vi "Go.vi"(6 "assembly type":string, 8 "First?":bool, 9 "Timing Data":T1(array[cluster]), 10 "Control In":T2={"I-O.lvclass"=refnum, "Gantry"=refnum, "Dispenser"="COM1"}, 11 "Sensor Dispense in":refnum<class "Sensor Dispense.lvclass">) -> (2 "Control Out":T2={"I-O.lvclass"=refnum, "Gantry"=refnum, "Dispenser"="COM1"}, 3 "Sensor Dispense out":refnum<class "Sensor Dispense.lvclass">)   [LabVIEW 2021, in "Sensor Dispense.lvclass"]
uses:
  Sensor Dispense.lvclass
  C:/Users/HEP/Documents/GitHub/Gantry/UCSB-Gantry-HEP-main/Classes/Routine/Dispense/Dispense.lvclass
  Classes/Controller/Controllers.ctl
  Classes/Controller/I-O/I-O.lvclass
  C:/Program Files (x86)/Aerotech/A3200/LabVIEW/2010/Bin/Aerotech.A3200.dll
  Program Files (x86)/Aerotech/A3200/LabVIEW/2010/Bin/Aerotech.A3200.dll
  Sensor Dispense.lvclass/Sensor Dispense.ctl
  Classes/Controller/Motion/Motion.lvclass
  Classes/Controller/Dispenser/Dispenser.lvclass
  Classes/Controller/Motion/A3200/A3200.lvclass
  Classes/Controller/Controller.lvclass
panel:
  out "error out":errorcluster
  in  "error in (no error)":errorcluster
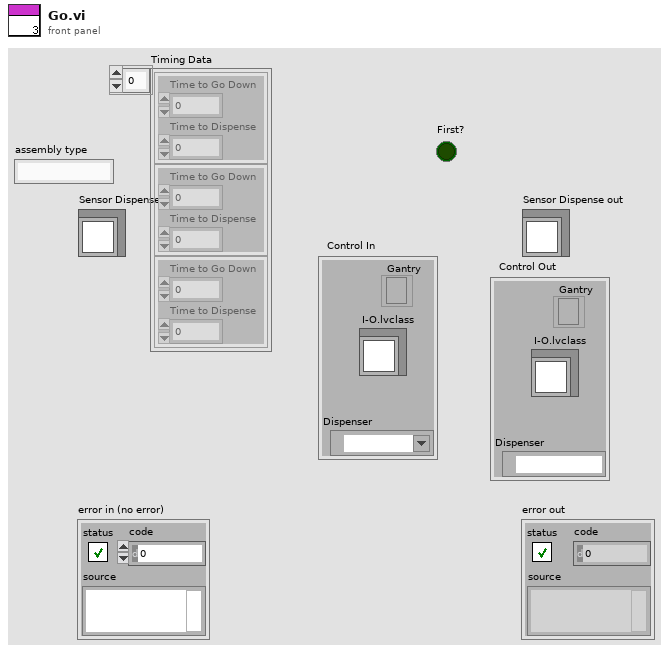
[diagram p1: front panel]
types:
  T1 = cluster{"Time to Go Down":i32, "Time to Dispense":i32}[]
  T2 = typedef "Controller.lvclass/Controllers.ctl" = cluster{"I-O.lvclass":refnum<class "I-O.lvclass">, "Gantry":refnum<k24>, "Dispenser":refnum<visa-resource-name>}
  T3 = cluster{"Endpoints":dbl[][], "Center":dbl[], "CW/CCW":dbl, "Dispense Type":enum16{"N-gon", "Square", "Arc", "Dot", "Line", "Circle"}}[]
  T4 = cluster{"Endpoints":dbl[][], "Center":dbl[], "CW/CCW":dbl, "Dispense Type":enum16{"N-gon", "Square", "Arc", "Dot", "Line", "Circle"}}
  T5 = enum16{"N-gon", "Square", "Arc", "Dot", "Line", "Circle"}
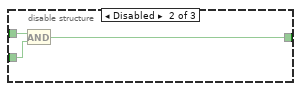
[diagram p3: hidden frame]
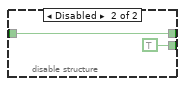
[diagram p4: hidden frame]
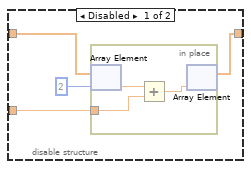
[diagram p6: hidden frame]
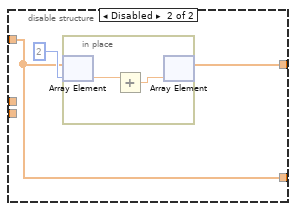
[diagram p7: hidden frame]
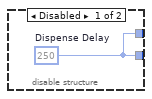
[diagram p9: hidden frame]
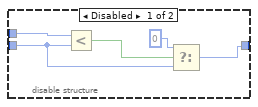
[diagram p10: hidden frame]
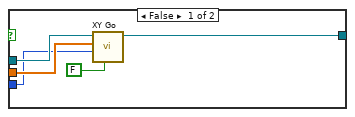
[diagram p11: hidden frame]
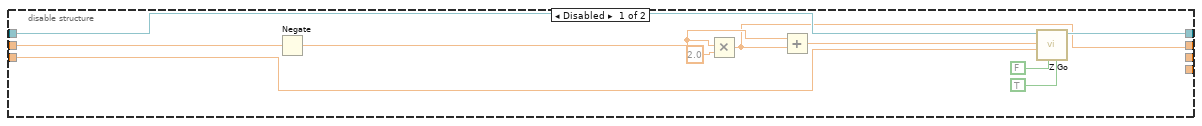
[diagram p12: hidden frame]
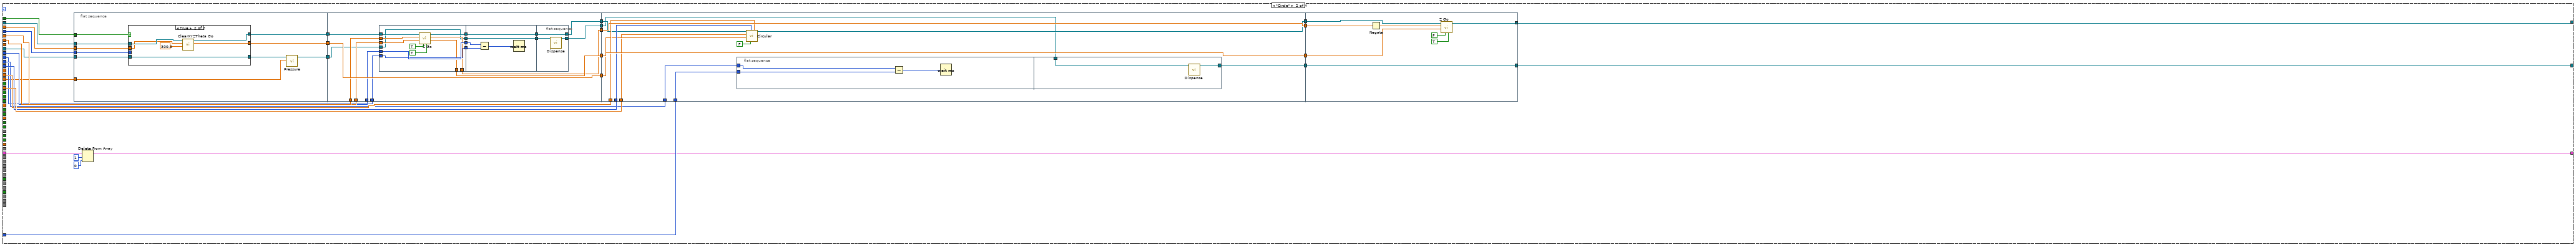
[diagram p14: hidden frame]
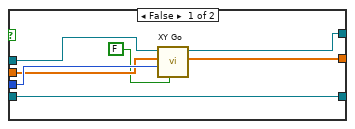
[diagram p15: hidden frame]
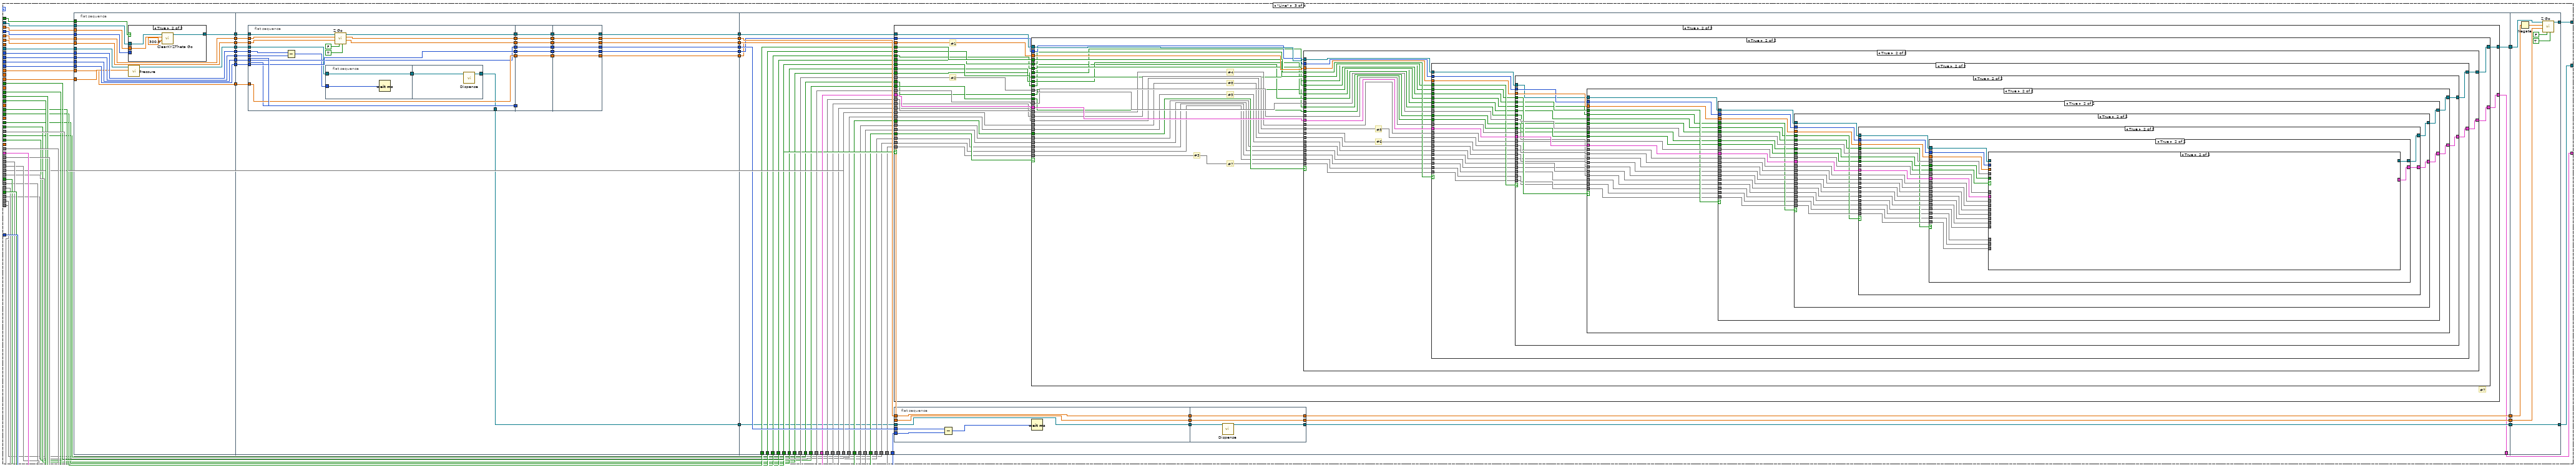
[diagram p16: hidden frame]
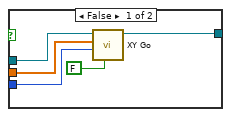
[diagram p17: hidden frame]
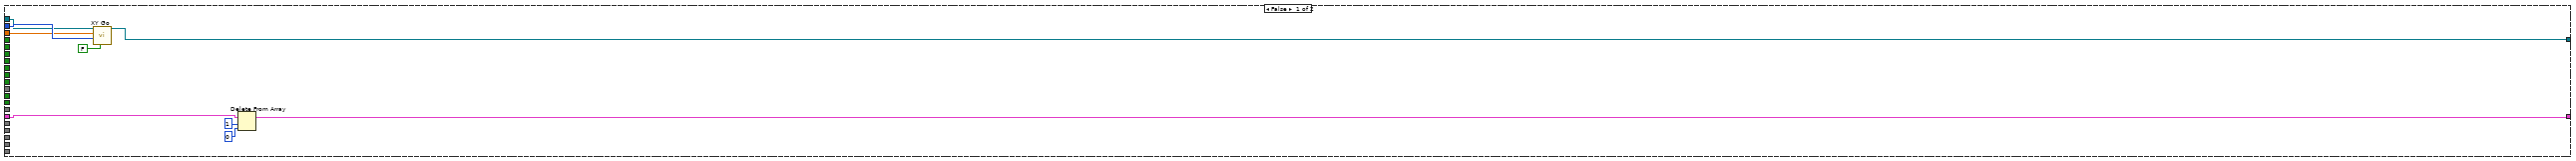
[diagram p18: hidden frame]
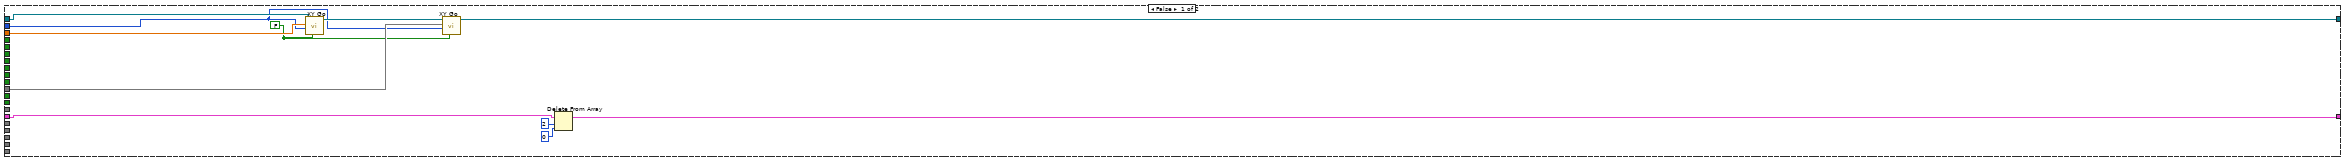
[diagram p19: hidden frame]
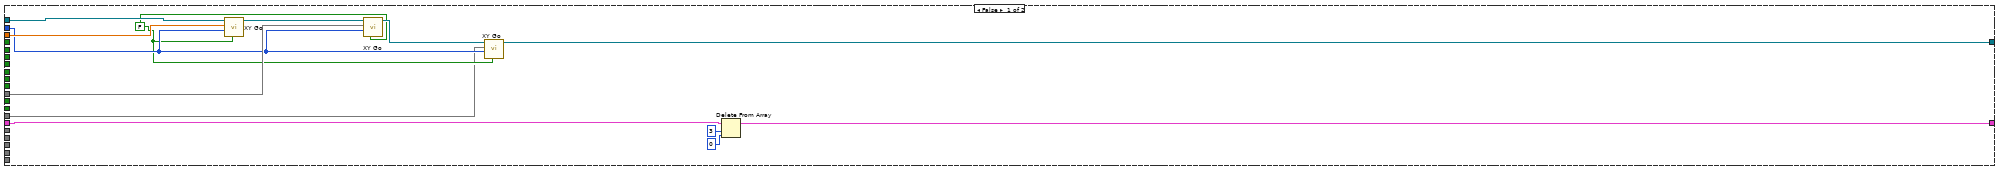
[diagram p20: hidden frame]
diagram:
  n1 = case shown="No Error" "error in (no error)" {
    selector: "error in (no error)" -> [w9 w1467]
    tunnel: "Sensor Dispense in" -> [w14 w1466]
    tunnel: [w13 w1466] -> w6
    tunnel: "Control In" -> [w12 w1465]
    tunnel: [w11 w1465] -> w4
    tunnel: [w10 w1467] -> w3
    tunnel: "First?" -> [w8 _]
    frame No Error {
      n2 = in-place {
        in-place-border: w14 -> [w27]
        in-place-border: [w26] -> w13
        in-place-border: w9 -> [w20]
        in-place-border: [w19] -> w10
        in-place-border: w8 -> [w15]
        n3 = in-place-cluster #1(w12) -> ("Gantry"=w28:refnum<k24>, "Dispenser"=w23:refnum<visa-resource-name>)
        n4 = Unbundle By Name(w27) -> ("Dispense Steps"=w24:T3, "Glue Speed"=w18:i32, "Move Speed"=w29:i32, "Line Pressure"=w16:dbl, "Dot Pressure"=w17:dbl)
        n5 = while {
          tunnel: w29 -> [w180]
          shift-right: [w174] -> w25
          shift-left: w28 -> [w43]
          tunnel: w18 -> [w179]
          shift-right: [w167] -> w26
          shift-left: w27 -> [w177]
          shift-right: [w169] -> w21
          shift-left: w23 -> [w172]
          tunnel: "Timing Data" -> [w171] mode=indexing
          shift-right: [w42] -> w19
          shift-left: w20 -> [w41]
          tunnel: w17 -> [w165]
          tunnel: w16 -> [w164]
          shift-right: [w128] -> _
          shift-left: w24 -> [w80]
          tunnel: w15 -> [w30]
          i -> [w176]
          stop <- w130 stop-if-true
          # "740 is good"
          # "compares 3 and 4"
          # "compares 2 and 3"
          # "Compares 1 and 2"
          # "#2"
          # "#3"
          # "#4"
          # "#3"
          # "1/11/23 - Originally 750"
          n6 = call "get Estop status.vi"("error in (no error)"=w41, "controller in"=w43) -> ("error out"=w42:errorcluster, "Estop?"=w40:bool, "controller out"=w36:refnum<k24>)  [unwired: 7 in]
          n7 = Equal To 0?(x=w176) -> (x = 0?=w31:bool)
          n8 = disable-structure shown="Enabled" {
            disable-tunnel: [w182 w185 w190] -> w32
            disable-tunnel: w31 -> [w182 w184 w191]
            disable-tunnel: w30 -> [w181 w183 w186]
            frame Disabled {
            }
            frame Disabled {
              n9 = And(x=w184, y=w183) -> (x .and. y?=w185:bool)
            }
            frame Enabled {
              n10 = disable-structure shown="Enabled" {
                disable-tunnel: [w194 TRUE ("protomodule? (T)")] -> w188
                disable-tunnel: [TRUE ("element") w195] -> w187
                disable-tunnel: w186 -> [_ w195]
                frame Enabled {
                  n11 = call "protomodule or module.vi"("assembly type"="assembly type") -> ("protomodule? (T)"=w194:bool)  [unwired: 10 in]
                }
                frame Disabled {
                }
              }
              n12 = Build Array(w191, w187, w188) -> (w189:bool[])
              n13 = And Array Elements(Boolean array=w189) -> (logical AND=w190:bool)
            }
          }
          n14 = Stop(stop? (T)=w40) -> ()
          n15 = Index Array(array=w80, index=6) -> (element=w123:T4)
          n16 = Index Array(array=w80, index=7) -> (element=w121:T4)
          n17 = Unbundle By Name(w123) -> ("Endpoints"=w122:dbl[][])  [unwired: 1 out]
          n18 = Unbundle By Name(w121) -> ("Endpoints"=w120:dbl[][])  [unwired: 1 out]
          n19 = Index Array(array=w122) -> (element #1=w105:dbl[], element #2=w46:dbl[])  [unwired: 4 in]
          n20 = Index Array(array=w120) -> (element #1=w99:dbl[], element #2=w78:dbl[])  [unwired: 4 in]
          n21 = Equal?(x=w46, y=w99) -> (x = y?=w100:bool[])
          n22 = Index Array(array=w80) -> (element=w160:T4)  [unwired: 1 in]
          n23 = Index Array(array=w100) -> (element #1=w98:bool, element #2=w97:bool)  [unwired: 2 in]
          n24 = And(x=w98, y=w97) -> (x .and. y?=w96:bool)
          n25 = Unbundle By Name(w160) -> ("Endpoints"=w151:dbl[][], "Center"=w173:dbl[], "Dispense Type"=w175:T5, "CW/CCW"=w178:dbl)
          n26 = property on="Property Node" class="Sensor Dispense.lvclass"(reference=w177) -> (reference out=w167:refnum<class "Sensor Dispense.lvclass">, "Z height"=w37:dbl, "Z speed"=w168:dbl, "Tip Height"=w34:dbl)  [unwired: 1 in, 1 out]
          n27 = Index Array(array=w151) -> (element #2=w150:dbl[])  [unwired: 4 in, 1 out]
          n28 = Index Array(array=w151) -> (element #1=w38:dbl[], element #2=w39:dbl[])  [unwired: 4 in]
          n29 = disable-structure shown="Enabled" {
            disable-tunnel: w36 -> [w203 w243]
            disable-tunnel: w38 -> [w197 w242]
            disable-tunnel: [w202 w243] -> w35
            disable-tunnel: w37 -> [w198 _]
            disable-tunnel: w32 -> [w201 _]
            disable-tunnel: w34 -> [w200 _]
            disable-tunnel: [w199 w242] -> w33
            frame Enabled {
              n30 = case shown="True" w201 {
                tunnel: w203 -> [w205 w214]
                tunnel: [w205 w209] -> w202
                tunnel: w200 -> [_ w206]
                tunnel: [w204 w210] -> w199
                tunnel: w198 -> [_ w208]
                tunnel: w197 -> [w204 w207]
                frame False {
                }
                frame True {
                  n31 = disable-structure shown="Enabled" {
                    disable-tunnel: [w220 w234] -> w213
                    disable-tunnel: [w219 w235] -> w210
                    disable-tunnel: w208 -> [w218 _]
                    disable-tunnel: w207 -> [w216 w235]
                    disable-tunnel: w206 -> [w215 _]
                    frame Enabled {
                      n32 = disable-structure shown="Enabled" {
                        disable-tunnel: [w224 w228] -> w219
                        disable-tunnel: w216 -> [w222 w228]
                        disable-tunnel: w215 -> [w221 _]
                        frame Disabled {
                          n33 = in-place {
                            in-place-border: w221 -> [w226]
                            n34 = in-place-array #2(w222, 2) -> (w227:dbl)
                            n35 = Add(x=w227, y=w226) -> (x+y=w225:dbl)
                            n36 = in-place-array #2(w225) -> (w224:dbl[])  [unwired: 1 out]
                          }
                        }
                        frame Enabled {
                        }
                      }
                      n37 = in-place {
                        in-place-border: w218 -> [w232]
                        in-place-border: w215 -> [w230]
                        n38 = in-place-array #3(w216, 2) -> (w233:dbl)
                        n39 = Negate(x=w230) -> (-x=w229:dbl)
                        n40 = Compound Arithmetic op=ADD(w233, w232, w229) -> (w231:dbl)
                        n41 = in-place-array #3(w231) -> (w220:dbl[])  [unwired: 1 out]
                      }
                    }
                    frame Disabled {
                      n42 = in-place {
                        n43 = in-place-array #4(w235, 2) -> (w238:dbl)
                        n44 = Add(x=w238) -> (x+y=w237:dbl)  [unwired: 1 in]
                        n45 = in-place-array #4(w237) -> (w234:dbl[])  [unwired: 1 out]
                      }
                    }
                  }
                  n46 = call "ClearXYZTheta Go.vi"("Speed"=300.0, "XYZTheta In"=w213, "Gantry In"=w214) -> ("error out"=w212:errorcluster, "Gantry Out"=w209:refnum<k24>)  [unwired: 6 in, 1 out]
                  n47 = while {
                    shift-right: [w239] -> _
                    shift-left: w212 -> [w240]
                    stop <- w241 stop-if-true
                    n48 = call "Prompt User for Input"("error in (no error)"=w240) -> ("Tip on component?"=w241:bool, "error out"=w239:errorcluster)  [unwired: 16 in, 1 out]
                  }
                }
              }
            }
            frame Disabled {
            }
          }
          n49 = Unbundle By Name(w171) -> ("Time to Go Down"=w170:i32, "Time to Dispense"=w162:i32)
          n50 = disable-structure shown="Enabled" {
            disable-tunnel: [w244 w248] -> w166
            disable-tunnel: [w244 w246] -> w163
            disable-tunnel: w162 -> [_ w247]
            frame Disabled {
              w244 = 250  # Dispense Delay
            }
            frame Enabled {
              w245 = 450  # End Dispense Delay
              w248 = 740  # Start Dispense Delay
              # "For arcs it is set to 250"
              # "525 - 1/23/2023"
              # "Originally 0"
              n51 = disable-structure shown="Enabled" {
                disable-tunnel: w247 -> [w253 _]
                disable-tunnel: [w250 w254] -> w246
                disable-tunnel: w245 -> [w249 w254]
                frame Disabled {
                  n52 = Less?(x=w253, y=w249) -> (x < y?=w252:bool)
                  n53 = Select(t=0, s=w252, f=w249) -> (s? t:f=w250:i32)
                }
                frame Enabled {
                }
              }
            }
          }
          n54 = Index Array(array=w80, index=2) -> (element=w157:T4)
          n55 = Index Array(array=w80, index=1) -> (element=w159:T4)
          n56 = Unbundle By Name(w157) -> ("Endpoints"=w154:dbl[][], "Center"=w135:dbl[])
          n57 = Unbundle By Name(w159) -> ("Endpoints"=w158:dbl[][], "Center"=w136:dbl[])
          n58 = Index Array(array=w80, index=3) -> (element=w156:T4)
          n59 = Unbundle By Name(w156) -> ("Endpoints"=w155:dbl[][], "Center"=w134:dbl[])
          n60 = Index Array(array=w154) -> (element #1=w148:dbl[], element #2=w44:dbl[])  [unwired: 4 in]
          n61 = Index Array(array=w158) -> (element #1=w149:dbl[], element #2=w137:dbl[])  [unwired: 4 in]
          n62 = Equal?(x=w150, y=w149) -> (x = y?=w146:bool[])
          n63 = Equal?(x=w137, y=w148) -> (x = y?=w143:bool[])
          n64 = Index Array(array=w155) -> (element #1=w147:dbl[], element #2=w45:dbl[])  [unwired: 4 in]
          n65 = Index Array(array=w80, index=10) -> (element=w89:T4)
          n66 = Index Array(array=w80, index=11) -> (element=w86:T4)
          n67 = Index Array(array=w80, index=12) -> (element=w83:T4)
          n68 = Equal?(x=w44, y=w147) -> (x = y?=w142:bool[])
          n69 = Index Array(array=w146) -> (element #1=w145:bool, element #2=w144:bool)  [unwired: 2 in]
          n70 = Index Array(array=w143) -> (element #1=w141:bool, element #2=w140:bool)  [unwired: 2 in]
          n71 = Index Array(array=w80, index=8) -> (element=w95:T4)
          n72 = Index Array(array=w80, index=9) -> (element=w92:T4)
          n73 = Index Array(array=w80, index=5) -> (element=w125:T4)
          n74 = Index Array(array=w80, index=4) -> (element=w127:T4)
          n75 = Unbundle By Name(w89) -> ("Endpoints"=w88:dbl[][])  [unwired: 1 out]
          n76 = Unbundle By Name(w86) -> ("Endpoints"=w85:dbl[][])  [unwired: 1 out]
          n77 = Unbundle By Name(w83) -> ("Endpoints"=w82:dbl[][])  [unwired: 1 out]
          n78 = Unbundle By Name(w95) -> ("Endpoints"=w94:dbl[][])  [unwired: 1 out]
          n79 = Unbundle By Name(w92) -> ("Endpoints"=w91:dbl[][])  [unwired: 1 out]
          n80 = Unbundle By Name(w125) -> ("Endpoints"=w124:dbl[][])  [unwired: 1 out]
          n81 = Unbundle By Name(w127) -> ("Endpoints"=w126:dbl[][])  [unwired: 1 out]
          n82 = And(x=w145, y=w144) -> (x .and. y?=w133:bool)
          n83 = Index Array(array=w142) -> (element #1=w139:bool, element #2=w138:bool)  [unwired: 2 in]
          n84 = And(x=w141, y=w140) -> (x .and. y?=w132:bool)
          n85 = And(x=w139, y=w138) -> (x .and. y?=w131:bool)
          n86 = Index Array(array=w88) -> (element #1=w67:dbl[], element #2=w61:dbl[])  [unwired: 4 in]
          n87 = Index Array(array=w85) -> (element #1=w60:dbl[], element #2=w55:dbl[])  [unwired: 4 in]
          n88 = Index Array(array=w82) -> (element #1=w54:dbl[], element #2=w49:dbl[])  [unwired: 4 in]
          n89 = Index Array(array=w94) -> (element #1=w79:dbl[], element #2=w72:dbl[])  [unwired: 4 in]
          n90 = Index Array(array=w91) -> (element #1=w73:dbl[], element #2=w66:dbl[])  [unwired: 4 in]
          n91 = Index Array(array=w124) -> (element #1=w110:dbl[], element #2=w48:dbl[])  [unwired: 4 in]
          n92 = Index Array(array=w126) -> (element #1=w115:dbl[], element #2=w47:dbl[])  [unwired: 4 in]
          n93 = Equal?(x=w61, y=w60) -> (x = y?=w59:bool[])
          n94 = Equal?(x=w48, y=w105) -> (x = y?=w104:bool[])
          n95 = Equal?(x=w55, y=w54) -> (x = y?=w53:bool[])
          n96 = Equal?(x=w66, y=w67) -> (x = y?=w65:bool[])
          n97 = Equal?(x=w72, y=w73) -> (x = y?=w71:bool[])
          n98 = Equal?(x=w47, y=w110) -> (x = y?=w109:bool[])
          n99 = Equal?(x=w78, y=w79) -> (x = y?=w77:bool[])
          n100 = Equal?(x=w45, y=w115) -> (x = y?=w114:bool[])
          n101 = Index Array(array=w59) -> (element #1=w58:bool, element #2=w57:bool)  [unwired: 2 in]
          n102 = Index Array(array=w104) -> (element #1=w103:bool, element #2=w102:bool)  [unwired: 2 in]
          n103 = Index Array(array=w53) -> (element #1=w52:bool, element #2=w51:bool)  [unwired: 2 in]
          n104 = Index Array(array=w65) -> (element #1=w64:bool, element #2=w63:bool)  [unwired: 2 in]
          n105 = Index Array(array=w71) -> (element #1=w70:bool, element #2=w69:bool)  [unwired: 2 in]
          n106 = Index Array(array=w109) -> (element #1=w108:bool, element #2=w107:bool)  [unwired: 2 in]
          n107 = Index Array(array=w77) -> (element #1=w76:bool, element #2=w75:bool)  [unwired: 2 in]
          n108 = Index Array(array=w114) -> (element #1=w113:bool, element #2=w112:bool)  [unwired: 2 in]
          n109 = And(x=w58, y=w57) -> (x .and. y?=w56:bool)
          n110 = And(x=w103, y=w102) -> (x .and. y?=w101:bool)
          n111 = And(x=w52, y=w51) -> (x .and. y?=w50:bool)
          n112 = And(x=w64, y=w63) -> (x .and. y?=w62:bool)
          n113 = And(x=w70, y=w69) -> (x .and. y?=w68:bool)
          n114 = And(x=w108, y=w107) -> (x .and. y?=w106:bool)
          n115 = And(x=w76, y=w75) -> (x .and. y?=w74:bool)
          n116 = And(x=w113, y=w112) -> (x .and. y?=w111:bool)
          n117 = case shown="\"Dot\", Default" w175 {
            tunnel: w173 -> [_ w408 _ w1258]
            tunnel: w35 -> [w284 w409 w501 w1264]
            tunnel: w180 -> [w269 w402 w559 w1263]
            tunnel: [w283 w412 w557 w1254] -> w174
            tunnel: w179 -> [_ w407 w551 w1257]
            tunnel: w178 -> [_ w406 _ w1256]
            tunnel: w168 -> [w277 w404 w548 w1259]
            tunnel: w37 -> [w278 w405 w549 w1260]
            tunnel: w31 -> [w285 w403 w498 w1265]
            tunnel: w172 -> [w276 w388 w554 w1250]
            tunnel: w170 -> [w274 w393 w552 w1262]
            tunnel: w162 -> [w279 w394 w550 w1255]
            tunnel: w166 -> [w280 w392 w553 w1261]
            tunnel: [w282 w389 w555 w1253] -> w169
            tunnel: w165 -> [w268 _ _ _]
            tunnel: w164 -> [_ w386 w531 w1249]
            tunnel: w163 -> [_ w385 w530 w1248]
            tunnel: w137 -> [_ _ w527 w1247]
            tunnel: w136 -> [_ _ _ w1246]
            tunnel: w135 -> [_ _ _ w1245]
            tunnel: w134 -> [_ _ _ w1244]
            tunnel: w45 -> [_ _ w522 w1243]
            tunnel: w133 -> [_ _ w525 w1242]
            tunnel: w132 -> [_ _ w524 w1241]
            tunnel: w131 -> [_ _ w523 w1240]
            tunnel: w80 -> [w260 w384 w528 w1239]
            tunnel: [w257 w381 w529 w1238] -> w128
            tunnel: w44 -> [_ _ w526 w1237]
            tunnel: w111 -> [_ _ w521 _]
            tunnel: w47 -> [_ _ w520 _]
            tunnel: w106 -> [_ _ w519 _]
            tunnel: w48 -> [_ _ w518 _]
            tunnel: w101 -> [_ _ w517 _]
            tunnel: w96 -> [_ _ w516 _]
            tunnel: w46 -> [_ _ w515 _]
            tunnel: w78 -> [_ _ w514 _]
            tunnel: w74 -> [_ _ w513 _]
            tunnel: w72 -> [_ _ w512 _]
            tunnel: w68 -> [_ _ w511 _]
            tunnel: w66 -> [_ _ w510 _]
            tunnel: w62 -> [_ _ w509 _]
            tunnel: w61 -> [_ _ w508 _]
            tunnel: w56 -> [_ _ w507 _]
            tunnel: w55 -> [_ _ w506 _]
            tunnel: w50 -> [_ _ w505 _]
            tunnel: w49 -> [_ _ w504 _]
            tunnel: w33 -> [w255 w380 w500 w1236]
            tunnel: w39 -> [_ _ w499 w1235]
            frame "Dot", Default {
              n118 = flat-sequence {
                tunnel: w285 -> [w286]
                tunnel: w284 -> [w297]
                tunnel: w255 -> [w296]
                tunnel: [w295] -> w281
                tunnel: w280 -> [w292]
                tunnel: w279 -> [_]
                tunnel: w278 -> [w294]
                tunnel: w277 -> [w291]
                tunnel: w276 -> [w289]
                tunnel: [w294] -> w275
                tunnel: w274 -> [w293]
                tunnel: [w293] -> w273
                tunnel: [w292] -> w272
                tunnel: [w288] -> w271
                tunnel: [w291] -> w270
                tunnel: w269 -> [w290]
                tunnel: w268 -> [w287]
                tunnel: [w324] -> w265
                tunnel: w281 -> [w323]
                tunnel: [w320] -> w264
                tunnel: w275 -> [w319]
                tunnel: w273 -> [w318]
                tunnel: w272 -> [w317]
                tunnel: w271 -> [w316]
                tunnel: w270 -> [w313]
                tunnel: [w311] -> w263
                tunnel: [w310] -> w262
                tunnel: w265 -> [w352]
                tunnel: w264 -> [w351]
                tunnel: w263 -> [w350]
                tunnel: w262 -> [w349]
                tunnel: [w353] -> w267
                tunnel: [w352] -> w266
                tunnel: [w347] -> w261
                tunnel: [w348] -> w256
                tunnel: [w367] -> w282
                tunnel: [w370] -> w283
                tunnel: w267 -> [w371]
                tunnel: w266 -> [w367]
                tunnel: w261 -> [w369]
                tunnel: w256 -> [w368]
                frame #0 {
                  n119 = case shown="True" w286 {
                    tunnel: w297 -> [w302 w306]
                    tunnel: [w301 w305] -> w295
                    tunnel: w296 -> [w300 w304]
                    tunnel: w290 -> [w299 _]
                    frame False {
                      n120 = call "XY Go.vi"("return immediately"=FALSE, "Speed"=w299, "XY In"=w300, "Gantry In"=w302) -> ("Gantry Out"=w301:refnum<k24>)  [unwired: 5 in, 2 out]
                    }
                    frame True {
                      n121 = call "ClearXYZTheta Go.vi"("Speed"=300.0, "XYZTheta In"=w304, "Gantry In"=w306) -> ("Gantry Out"=w305:refnum<k24>)  [unwired: 6 in, 2 out]
                    }
                  }
                  n122 = call "Pressure.vi"("Pressure"=w287, "VISA resource name"=w289) -> ("VISA resource name out"=w288:refnum<visa-resource-name>)  [unwired: 8 in, 1 out]
                }
                frame #1 {
                  n123 = flat-sequence {
                    tunnel: w323 -> [w333]
                    tunnel: [w332] -> w321
                    tunnel: w319 -> [w326]
                    tunnel: w316 -> [w330]
                    tunnel: [w330] -> w315
                    tunnel: w313 -> [w329]
                    tunnel: [w328] -> w308
                    tunnel: [w325] -> w307
                    tunnel: [w340] -> w322
                    tunnel: w321 -> [w340]
                    tunnel: w318 -> [w339]
                    tunnel: w317 -> [w335]
                    tunnel: w315 -> [w338]
                    tunnel: [w338] -> w314
                    tunnel: [w337] -> w312
                    tunnel: [w336] -> w309
                    tunnel: w308 -> [w336]
                    tunnel: w307 -> [w337]
                    tunnel: [w346] -> w324
                    tunnel: w322 -> [w345]
                    tunnel: [w345] -> w320
                    tunnel: w314 -> [w344]
                    tunnel: w312 -> [w342]
                    tunnel: [w342] -> w311
                    tunnel: [w341] -> w310
                    tunnel: w309 -> [w341]
                    frame #0 {
                      n124 = call "Z Go.vi"("Increment"=TRUE, "Return Immediately"=TRUE, "Speed In"=w329, "Position In"=w326, "Gantry In"=w333) -> ("Speed Out"=w328:dbl, "Position Out"=w325:dbl, "Gantry Out"=w332:refnum<k24>)  [unwired: 3 in, 1 out]
                    }
                    frame #1 {
                      n125 = Subtract(x=w339, y=w335) -> (x-y=w334:i32)
                      n126 = Wait (ms)(milliseconds to wait=w334) -> ()  [unwired: 1 out]
                    }
                    frame #2 {
                      n127 = call "Dispense.vi"("Dispenser In"=w344) -> ("Dispenser Out"=w343:refnum<visa-resource-name>)  [unwired: 9 in, 1 out]
                      n128 = call "Dispense.vi"("Dispenser In"=w343) -> ("Dispenser Out"=w346:refnum<visa-resource-name>)  [unwired: 9 in, 1 out]
                    }
                  }
                }
                frame #2 {
                  n129 = disable-structure shown="Enabled" {
                    disable-tunnel: [w363 w366] -> w353
                    disable-tunnel: w351 -> [w362 w366]
                    disable-tunnel: w350 -> [w361 w364]
                    disable-tunnel: w349 -> [w358 w365]
                    disable-tunnel: [w354 _] -> _
                    disable-tunnel: [_ w365] -> w348
                    disable-tunnel: [_ w364] -> w347
                    frame Disabled {
                      n130 = Negate(x=w361) -> (-x=w356:dbl)
                      n131 = Multiply(x=w356, y=2.0) -> (x*y=w354:dbl)
                      n132 = Add(x=w356, y=w354) -> (x+y=w357:dbl)
                      n133 = call "Z Go.vi"("Increment"=TRUE, "Return Immediately"=FALSE, "Speed In"=w358, "Position In"=w357, "Gantry In"=w362) -> ("Gantry Out"=w363:refnum<k24>)  [unwired: 3 in, 3 out]
                    }
                    frame Enabled {
                    }
                  }
                }
                frame #3 {
                  n134 = disable-structure shown="Enabled" {
                    disable-tunnel: w371 -> [w378 w379]
                    disable-tunnel: [w377 w379] -> w370
                    disable-tunnel: w369 -> [w372 _]
                    disable-tunnel: w368 -> [w373 _]
                    frame Enabled {
                      n135 = Negate(x=w372) -> (-x=w376:dbl)
                      n136 = call "Z Go.vi"("Increment"=TRUE, "Return Immediately"=FALSE, "Speed In"=w373, "Position In"=w376, "Gantry In"=w378) -> ("Gantry Out"=w377:refnum<k24>)  [unwired: 3 in, 3 out]
                    }
                    frame Disabled {
                    }
                  }
                }
              }
              n137 = Delete From Array(array=w260, length=1, index=0) -> (array with subset deleted=w257:T3)  [unwired: 1 out]
            }
            frame "Circle" {
              n138 = flat-sequence {
                tunnel: [w421] -> w411
                tunnel: w409 -> [w422]
                tunnel: w403 -> [w413]
                tunnel: w402 -> [w420]
                tunnel: [w419] -> w400
                tunnel: w380 -> [w418]
                tunnel: w388 -> [w417]
                tunnel: [w415] -> w387
                tunnel: w386 -> [w414]
                tunnel: w405 -> [w445]
                tunnel: w404 -> [w446]
                tunnel: [w452] -> w401
                tunnel: [w443] -> w399
                tunnel: [w444] -> w398
                tunnel: w400 -> [w452]
                tunnel: w411 -> [w442]
                tunnel: [w451] -> w395
                tunnel: w393 -> [w450]
                tunnel: w392 -> [w449]
                tunnel: [w439] -> w391
                tunnel: w387 -> [w438]
                tunnel: [w474] -> w410
                tunnel: [w484] -> w397
                tunnel: [w483] -> w396
                tunnel: w394 -> [w482]
                tunnel: w395 -> [w472]
                tunnel: w401 -> [w477]
                tunnel: w399 -> [w484]
                tunnel: w398 -> [w483]
                tunnel: w406 -> [w480]
                tunnel: w407 -> [w478]
                tunnel: w408 -> [w476]
                tunnel: w391 -> [w475]
                tunnel: [w481] -> w390
                tunnel: w385 -> [w473]
                tunnel: [w495] -> w412
                tunnel: w410 -> [w496]
                tunnel: w397 -> [w497]
                tunnel: w396 -> [w494]
                tunnel: w390 -> [w493]
                tunnel: [w493] -> w389
                frame #0 {
                  n139 = case shown="True" w413 {
                    tunnel: w422 -> [w429 w435]
                    tunnel: [w428 w434] -> w421
                    tunnel: w420 -> [w427 _]
                    tunnel: [w426 w432] -> w419
                    tunnel: w418 -> [w425 w433]
                    tunnel: w417 -> [w424 w431]
                    tunnel: [w424 w431] -> w416
                    frame False {
                      n140 = call "XY Go.vi"("return immediately"=FALSE, "Speed"=w427, "XY In"=w425, "Gantry In"=w429) -> ("XY Out"=w426:dbl[], "Gantry Out"=w428:refnum<k24>)  [unwired: 5 in, 1 out]
                    }
                    frame True {
                      n141 = call "ClearXYZTheta Go.vi"("Speed"=300.0, "XYZTheta In"=w433, "Gantry In"=w435) -> ("XYZTheta Out"=w432:dbl[], "Gantry Out"=w434:refnum<k24>)  [unwired: 6 in, 1 out]
                    }
                  }
                  n142 = call "Pressure.vi"("Pressure"=w414, "VISA resource name"=w416) -> ("VISA resource name out"=w415:refnum<visa-resource-name>)  [unwired: 8 in, 1 out]
                }
                frame #1 {
                  n143 = flat-sequence {
                    tunnel: w449 -> [w462]
                    tunnel: w450 -> [w463]
                    tunnel: [w463] -> w448
                    tunnel: [w462] -> w447
                    tunnel: w446 -> [w461]
                    tunnel: w445 -> [w460]
                    tunnel: [w459] -> w444
                    tunnel: [w458] -> w443
                    tunnel: w442 -> [w457]
                    tunnel: [w456] -> w441
                    tunnel: w438 -> [w454]
                    tunnel: [w454] -> w437
                    tunnel: w448 -> [w468]
                    tunnel: w447 -> [w467]
                    tunnel: w441 -> [w466]
                    tunnel: [w466] -> w440
                    tunnel: w437 -> [w465]
                    tunnel: [w465] -> w436
                    tunnel: [w471] -> w451
                    tunnel: w440 -> [w470]
                    tunnel: [w470] -> w439
                    tunnel: w436 -> [w469]
                    frame #0 {
                      n144 = call "Z Go.vi"("Increment"=TRUE, "Return Immediately"=TRUE ("return immediately"), "Speed In"=w461, "Position In"=w460, "Gantry In"=w457) -> ("Speed Out"=w459:dbl, "Position Out"=w458:dbl, "Gantry Out"=w456:refnum<k24>)  [unwired: 3 in, 1 out]
                    }
                    frame #1 {
                      n145 = Subtract(x=w468, y=w467) -> (x-y=w464:i32)
                      n146 = Wait (ms)(milliseconds to wait=w464) -> ()  [unwired: 1 out]
                    }
                    frame #2 {
                      n147 = call "Dispense.vi"("Dispenser In"=w469) -> ("Dispenser Out"=w471:refnum<visa-resource-name>)  [unwired: 9 in, 1 out]
                    }
                  }
                }
                frame #2 {
                  n148 = flat-sequence {
                    tunnel: w482 -> [w487]
                    tunnel: w473 -> [w485]
                    tunnel: [w489] -> w481
                    tunnel: w472 -> [w488]
                    frame #0 {
                      n149 = Subtract(x=w487, y=w485) -> (x-y=w486:i32)
                      n150 = Wait (ms)(milliseconds to wait=w486) -> ()  [unwired: 1 out]
                    }
                    frame #1 {
                      n151 = call "Dispense.vi"("Dispenser In"=w488) -> ("Dispenser Out"=w489:refnum<visa-resource-name>)  [unwired: 9 in, 1 out]
                    }
                  }
                  n152 = call "Circular.vi"("Direction"=w480, "return immediately"=FALSE, "Speed"=w478, "XY End"=w477, "XY Center"=w476, "Gantry In"=w475) -> ("Gantry Out"=w474:refnum<k24>)  [unwired: 4 in, 1 out]
                }
                frame #3 {
                  n153 = Negate(x=w497) -> (-x=w492:dbl)
                  n154 = call "Z Go.vi"("Increment"=TRUE, "Return Immediately"=FALSE, "Speed In"=w494, "Position In"=w492, "Gantry In"=w496) -> ("Gantry Out"=w495:refnum<k24>)  [unwired: 3 in, 3 out]
                }
              }
              n155 = Delete From Array(array=w384, length=1, index=0) -> (array with subset deleted=w381:T3)  [unwired: 1 out]
            }
            frame "Line" {
              n156 = flat-sequence {
                tunnel: w501 -> [w574]
                tunnel: w559 -> [w573]
                tunnel: [w572] -> w558
                tunnel: w554 -> [w565]
                tunnel: w553 -> [w568]
                tunnel: w552 -> [w569]
                tunnel: w551 -> [w567]
                tunnel: w550 -> [w566]
                tunnel: w549 -> [w571]
                tunnel: w548 -> [w570]
                tunnel: [w571] -> w547
                tunnel: [w570] -> w546
                tunnel: [w569] -> w544
                tunnel: [w568] -> w543
                tunnel: [w564] -> w542
                tunnel: [w561] -> w540
                tunnel: [w567] -> w538
                tunnel: [w566] -> w536
                tunnel: w531 -> [w563]
                tunnel: w500 -> [w562]
                tunnel: w499 -> [w561]
                tunnel: w498 -> [w560]
                tunnel: w558 -> [w607]
                tunnel: w547 -> [w606]
                tunnel: w546 -> [w605]
                tunnel: [w602] -> w545
                tunnel: w544 -> [w599]
                tunnel: w543 -> [w600]
                tunnel: w542 -> [w601]
                tunnel: [w613] -> w541
                tunnel: w540 -> [w612]
                tunnel: [w611] -> w539
                tunnel: w538 -> [w610]
                tunnel: [w608] -> w537
                tunnel: w536 -> [w609]
                tunnel: [w604] -> w533
                tunnel: [w603] -> w503
                tunnel: [w584] -> w502
                tunnel: [w687] -> w556
                tunnel: w545 -> [w676]
                tunnel: w541 -> [w677]
                tunnel: w539 -> [w678]
                tunnel: w537 -> [w685]
                tunnel: [w675] -> w535
                tunnel: [w684] -> w534
                tunnel: w533 -> [w682]
                tunnel: [w681] -> w532
                tunnel: w530 -> [w674]
                tunnel: [w673] -> w529
                tunnel: w528 -> [w672]
                tunnel: w527 -> [w671]
                tunnel: w526 -> [w670]
                tunnel: w525 -> [w669]
                tunnel: w524 -> [w668]
                tunnel: w523 -> [w667]
                tunnel: w522 -> [w666]
                tunnel: w521 -> [w665]
                tunnel: w520 -> [w664]
                tunnel: w519 -> [w663]
                tunnel: w518 -> [w662]
                tunnel: w517 -> [w661]
                tunnel: w516 -> [w660]
                tunnel: w515 -> [w659]
                tunnel: w514 -> [w658]
                tunnel: w513 -> [w657]
                tunnel: w512 -> [w656]
                tunnel: w511 -> [w655]
                tunnel: w510 -> [w654]
                tunnel: w509 -> [w653]
                tunnel: w508 -> [w652]
                tunnel: w507 -> [w651]
                tunnel: w506 -> [w650]
                tunnel: w505 -> [w649]
                tunnel: w504 -> [w648]
                tunnel: w503 -> [w679]
                tunnel: w502 -> [w647]
                tunnel: [w1234] -> w557
                tunnel: w556 -> [w1233]
                tunnel: [w1233] -> w555
                tunnel: w535 -> [w1232]
                tunnel: w534 -> [w1231]
                tunnel: w532 -> [w1229]
                frame #0 {
                  n157 = case shown="True" w560 {
                    tunnel: w574 -> [w579 w583]
                    tunnel: w573 -> [w578 _]
                    tunnel: [w577 w582] -> w572
                    tunnel: w562 -> [w576 w581]
                    frame False {
                      n158 = call "XY Go.vi"("return immediately"=FALSE, "Speed"=w578, "XY In"=w576, "Gantry In"=w579) -> ("Gantry Out"=w577:refnum<k24>)  [unwired: 5 in, 2 out]
                    }
                    frame True {
                      n159 = call "ClearXYZTheta Go.vi"("Speed"=300.0, "XYZTheta In"=w581, "Gantry In"=w583) -> ("Gantry Out"=w582:refnum<k24>)  [unwired: 6 in, 2 out]
                    }
                  }
                  n160 = call "Pressure.vi"("Pressure"=w563, "VISA resource name"=w565) -> ("VISA resource name out"=w564:refnum<visa-resource-name>)  [unwired: 8 in, 1 out]
                }
                frame #1 {
                  n161 = flat-sequence {
                    tunnel: w599 -> [w622]
                    tunnel: w600 -> [w614]
                    tunnel: w612 -> [w621]
                    tunnel: w610 -> [w620]
                    tunnel: w609 -> [w619]
                    tunnel: w607 -> [w630]
                    tunnel: w606 -> [w629]
                    tunnel: w605 -> [w628]
                    tunnel: w601 -> [w616]
                    tunnel: [w622] -> w598
                    tunnel: [w614] -> w597
                    tunnel: [w621] -> w596
                    tunnel: [w620] -> w595
                    tunnel: [w619] -> w594
                    tunnel: [w625] -> w593
                    tunnel: [w624] -> w592
                    tunnel: [w623] -> w591
                    tunnel: [w617] -> w584
                    tunnel: w598 -> [_]
                    tunnel: w597 -> [_]
                    tunnel: w596 -> [w640]
                    tunnel: w595 -> [w639]
                    tunnel: w594 -> [w638]
                    tunnel: w593 -> [w637]
                    tunnel: w592 -> [w636]
                    tunnel: w591 -> [w635]
                    tunnel: [w640] -> w590
                    tunnel: [w639] -> w589
                    tunnel: [w638] -> w588
                    tunnel: [w637] -> w587
                    tunnel: [w636] -> w586
                    tunnel: [w635] -> w585
                    tunnel: [w646] -> w613
                    tunnel: [w645] -> w611
                    tunnel: [w644] -> w608
                    tunnel: [w643] -> w604
                    tunnel: [w642] -> w603
                    tunnel: [w641] -> w602
                    tunnel: w590 -> [w646]
                    tunnel: w589 -> [w645]
                    tunnel: w588 -> [w644]
                    tunnel: w587 -> [w643]
                    tunnel: w586 -> [w642]
                    tunnel: w585 -> [w641]
                    frame #0 {
                      n162 = Subtract(x=w622, y=w614) -> (x-y=w618:i32)
                      n163 = flat-sequence {
                        tunnel: w618 -> [w632]
                        tunnel: w616 -> [w631]
                        tunnel: [w631] -> w615
                        tunnel: [w634] -> w617
                        tunnel: w615 -> [w633]
                        frame #0 {
                          n164 = Wait (ms)(milliseconds to wait=w632) -> ()  [unwired: 1 out]
                        }
                        frame #1 {
                          n165 = call "Dispense.vi"("Dispenser In"=w633) -> ("Dispenser Out"=w634:refnum<visa-resource-name>)  [unwired: 9 in, 1 out]
                        }
                      }
                      n166 = call "Z Go.vi"("Increment"=TRUE ("Return Immediately"), "Return Immediately"=FALSE ("Increment"), "Speed In"=w628, "Position In"=w629, "Gantry In"=w630) -> ("Speed Out"=w624:dbl, "Position Out"=w625:dbl, "Gantry Out"=w623:refnum<k24>)  [unwired: 3 in, 1 out]
                    }
                    frame #1 {
                    }
                    frame #2 {
                    }
                  }
                }
                frame #2 {
                  n167 = case shown="True" w669 {
                    tunnel: w678 -> [w696 w721]
                    tunnel: w677 -> [w695 w724]
                    tunnel: w676 -> [w694 w723]
                    tunnel: [w693 w720] -> w675
                    tunnel: [w690 w719] -> w673
                    tunnel: w672 -> [w691 w725]
                    tunnel: w671 -> [_ w722]
                    tunnel: w670 -> [_ w718]
                    tunnel: w668 -> [_ w717]
                    tunnel: w667 -> [_ w716]
                    tunnel: w666 -> [_ w715]
                    tunnel: w665 -> [_ w714]
                    tunnel: w664 -> [_ w713]
                    tunnel: w663 -> [_ w712]
                    tunnel: w662 -> [_ w711]
                    tunnel: w661 -> [_ w710]
                    tunnel: w660 -> [_ w709]
                    tunnel: w659 -> [_ w708]
                    tunnel: w658 -> [_ w707]
                    tunnel: w657 -> [_ w706]
                    tunnel: w656 -> [_ w705]
                    tunnel: w655 -> [_ w704]
                    tunnel: w654 -> [_ w703]
                    tunnel: w653 -> [_ w702]
                    tunnel: w652 -> [_ w701]
                    tunnel: w651 -> [_ w700]
                    tunnel: w650 -> [_ w699]
                    tunnel: w649 -> [_ w698]
                    tunnel: w648 -> [_ w697]
                    frame False {
                      n168 = call "XY Go.vi"("return immediately"=FALSE, "Speed"=w696, "XY In"=w695, "Gantry In"=w694) -> ("Gantry Out"=w693:refnum<k24>)  [unwired: 5 in, 2 out]
                      n169 = Delete From Array(array=w691, length=1, index=0) -> (array with subset deleted=w690:T3)  [unwired: 1 out]
                    }
                    frame True {
                      # "#7"
                      # "#2"
                      # "#1"
                      n170 = case shown="True" w717 {
                        tunnel: w725 -> [w736 w764]
                        tunnel: w724 -> [w733 w762]
                        tunnel: w723 -> [w732 w760]
                        tunnel: w722 -> [w730 w761]
                        tunnel: w721 -> [w729 w758]
                        tunnel: [w728 w759] -> w720
                        tunnel: [w727 w763] -> w719
                        tunnel: w718 -> [_ w757]
                        tunnel: w716 -> [_ w756]
                        tunnel: w715 -> [_ w755]
                        tunnel: w714 -> [_ w754]
                        tunnel: w713 -> [_ w753]
                        tunnel: w712 -> [_ w752]
                        tunnel: w711 -> [_ w751]
                        tunnel: w710 -> [_ w750]
                        tunnel: w709 -> [_ w749]
                        tunnel: w708 -> [_ w748]
                        tunnel: w707 -> [_ w747]
                        tunnel: w706 -> [_ w746]
                        tunnel: w705 -> [_ w745]
                        tunnel: w704 -> [_ w744]
                        tunnel: w703 -> [_ w743]
                        tunnel: w702 -> [_ w742]
                        tunnel: w701 -> [_ w741]
                        tunnel: w700 -> [_ w740]
                        tunnel: w699 -> [_ w739]
                        tunnel: w698 -> [_ w738]
                        tunnel: w697 -> [_ w737]
                        frame False {
                          w726 = FALSE ("return immediately")
                          n171 = call "XY Go.vi"("return immediately"=w726, "Speed"=w729, "XY In"=w733, "Gantry In"=w732) -> ("Gantry Out"=w731:refnum<k24>)  [unwired: 5 in, 2 out]
                          n172 = call "XY Go.vi"("return immediately"=w726, "Speed"=w729, "XY In"=w730, "Gantry In"=w731) -> ("Gantry Out"=w728:refnum<k24>)  [unwired: 5 in, 2 out]
                          n173 = Delete From Array(array=w736, length=2, index=0) -> (array with subset deleted=w727:T3)  [unwired: 1 out]
                        }
                        frame True {
                          # "#9"
                          # "#8"
                          # "#3"
                          # "#4"
                          # "#7"
                          n174 = case shown="True" w756 {
                            tunnel: w764 -> [w777 w798]
                            tunnel: [w774 w797] -> w763
                            tunnel: w762 -> [w773 w804]
                            tunnel: w761 -> [w772 w803]
                            tunnel: w760 -> [w771 w800]
                            tunnel: [w768 w799] -> w759
                            tunnel: w758 -> [w767 w801]
                            tunnel: w757 -> [w765 w802]
                            tunnel: w755 -> [_ w796]
                            tunnel: w754 -> [_ w795]
                            tunnel: w753 -> [_ w794]
                            tunnel: w752 -> [_ w793]
                            tunnel: w751 -> [_ w792]
                            tunnel: w750 -> [_ w791]
                            tunnel: w749 -> [_ w790]
                            tunnel: w748 -> [_ w789]
                            tunnel: w747 -> [_ w788]
                            tunnel: w746 -> [_ w787]
                            tunnel: w745 -> [_ w786]
                            tunnel: w744 -> [_ w785]
                            tunnel: w743 -> [_ w784]
                            tunnel: w742 -> [_ w783]
                            tunnel: w741 -> [_ w782]
                            tunnel: w740 -> [_ w781]
                            tunnel: w739 -> [_ w780]
                            tunnel: w738 -> [_ w779]
                            tunnel: w737 -> [_ w778]
                            frame False {
                              w766 = FALSE ("return immediately")
                              n175 = call "XY Go.vi"("return immediately"=w766, "Speed"=w767, "XY In"=w773, "Gantry In"=w771) -> ("Gantry Out"=w770:refnum<k24>)  [unwired: 5 in, 2 out]
                              n176 = call "XY Go.vi"("return immediately"=w766, "Speed"=w767, "XY In"=w772, "Gantry In"=w770) -> ("Gantry Out"=w769:refnum<k24>)  [unwired: 5 in, 2 out]
                              n177 = call "XY Go.vi"("return immediately"=w766, "Speed"=w767, "XY In"=w765, "Gantry In"=w769) -> ("Gantry Out"=w768:refnum<k24>)  [unwired: 5 in, 2 out]
                              n178 = Delete From Array(array=w777, length=3, index=0) -> (array with subset deleted=w774:T3)  [unwired: 1 out]
                            }
                            frame True {
                              # "#5"
                              # "#6"
                              n179 = case shown="True" w795 {
                                tunnel: w804 -> [w818 w842]
                                tunnel: w803 -> [w817 w841]
                                tunnel: w802 -> [w816 w840]
                                tunnel: w801 -> [w815 w838]
                                tunnel: w800 -> [w814 w837]
                                tunnel: [w810 w836] -> w799
                                tunnel: w798 -> [w807 w844]
                                tunnel: [w806 w843] -> w797
                                tunnel: w796 -> [w805 w839]
                                tunnel: w794 -> [_ w835]
                                tunnel: w793 -> [_ w834]
                                tunnel: w792 -> [_ w819]
                                tunnel: w791 -> [_ w833]
                                tunnel: w790 -> [_ w832]
                                tunnel: w789 -> [_ w831]
                                tunnel: w788 -> [_ w830]
                                tunnel: w787 -> [_ w829]
                                tunnel: w786 -> [_ w828]
                                tunnel: w785 -> [_ w827]
                                tunnel: w784 -> [_ w826]
                                tunnel: w783 -> [_ w825]
                                tunnel: w782 -> [_ w824]
                                tunnel: w781 -> [_ w823]
                                tunnel: w780 -> [_ w822]
                                tunnel: w779 -> [_ w821]
                                tunnel: w778 -> [_ w820]
                                frame False {
                                n180 = call "XY Go.vi"("Speed"=w815, "XY In"=w818, "Gantry In"=w814) -> ("Gantry Out"=w813:refnum<k24>)  [unwired: 6 in, 2 out]
                                n181 = call "XY Go.vi"("Speed"=w815, "XY In"=w817, "Gantry In"=w813) -> ("Gantry Out"=w812:refnum<k24>)  [unwired: 6 in, 2 out]
                                n182 = call "XY Go.vi"("Speed"=w815, "XY In"=w816, "Gantry In"=w812) -> ("Gantry Out"=w811:refnum<k24>)  [unwired: 6 in, 2 out]
                                n183 = call "XY Go.vi"("Speed"=w815, "XY In"=w805, "Gantry In"=w811) -> ("Gantry Out"=w810:refnum<k24>)  [unwired: 6 in, 2 out]
                                n184 = Delete From Array(array=w807, length=4, index=0) -> (array with subset deleted=w806:T3)  [unwired: 1 out]
                                }
                                frame True {
                                n185 = case shown="True" w834 {
                                tunnel: w844 -> [w860 w885]
                                tunnel: [w859 w884] -> w843
                                tunnel: w842 -> [w856 w883]
                                tunnel: w841 -> [w855 w882]
                                tunnel: w840 -> [w854 w880]
                                tunnel: w839 -> [w853 w879]
                                tunnel: w838 -> [w852 w878]
                                tunnel: w837 -> [w851 w877]
                                tunnel: [w846 w876] -> w836
                                tunnel: w835 -> [w845 w881]
                                tunnel: w819 -> [_ w875]
                                tunnel: w833 -> [_ w874]
                                tunnel: w832 -> [_ w873]
                                tunnel: w831 -> [_ w872]
                                tunnel: w830 -> [_ w871]
                                tunnel: w829 -> [_ w870]
                                tunnel: w828 -> [_ w869]
                                tunnel: w827 -> [_ w868]
                                tunnel: w826 -> [_ w867]
                                tunnel: w825 -> [_ w866]
                                tunnel: w824 -> [_ w865]
                                tunnel: w823 -> [_ w864]
                                tunnel: w822 -> [_ w863]
                                tunnel: w821 -> [_ w862]
                                tunnel: w820 -> [_ w861]
                                frame False {
                                n186 = call "XY Go.vi"("Speed"=w852, "XY In"=w856, "Gantry In"=w851) -> ("Gantry Out"=w850:refnum<k24>)  [unwired: 6 in, 2 out]
                                n187 = call "XY Go.vi"("Speed"=w852, "XY In"=w855, "Gantry In"=w850) -> ("Gantry Out"=w849:refnum<k24>)  [unwired: 6 in, 2 out]
                                n188 = call "XY Go.vi"("Speed"=w852, "XY In"=w854, "Gantry In"=w849) -> ("Gantry Out"=w848:refnum<k24>)  [unwired: 6 in, 2 out]
                                n189 = call "XY Go.vi"("Speed"=w852, "XY In"=w853, "Gantry In"=w848) -> ("Gantry Out"=w847:refnum<k24>)  [unwired: 6 in, 2 out]
                                n190 = call "XY Go.vi"("Speed"=w852, "XY In"=w845, "Gantry In"=w847) -> ("Gantry Out"=w846:refnum<k24>)  [unwired: 6 in, 2 out]
                                n191 = Delete From Array(array=w860, length=5, index=0) -> (array with subset deleted=w859:T3)  [unwired: 1 out]
                                }
                                frame True {
                                n192 = case shown="True" w874 {
                                tunnel: w885 -> [w901 w927]
                                tunnel: [w900 w926] -> w884
                                tunnel: w883 -> [w899 w925]
                                tunnel: w882 -> [w898 w924]
                                tunnel: w881 -> [w888 w923]
                                tunnel: w880 -> [w886 w922]
                                tunnel: w879 -> [w887 w920]
                                tunnel: w878 -> [w897 w919]
                                tunnel: w877 -> [w896 w918]
                                tunnel: [w890 w917] -> w876
                                tunnel: w875 -> [w889 w921]
                                tunnel: w873 -> [_ w916]
                                tunnel: w872 -> [_ w915]
                                tunnel: w871 -> [_ w914]
                                tunnel: w870 -> [_ w913]
                                tunnel: w869 -> [_ w912]
                                tunnel: w868 -> [_ w911]
                                tunnel: w867 -> [_ w910]
                                tunnel: w866 -> [_ w909]
                                tunnel: w865 -> [_ w908]
                                tunnel: w864 -> [_ w907]
                                tunnel: w863 -> [_ w906]
                                tunnel: w862 -> [_ w905]
                                tunnel: w861 -> [_ w904]
                                frame False {
                                n193 = call "XY Go.vi"("Speed"=w897, "XY In"=w899, "Gantry In"=w896) -> ("Gantry Out"=w895:refnum<k24>)  [unwired: 6 in, 2 out]
                                n194 = call "XY Go.vi"("Speed"=w897, "XY In"=w898, "Gantry In"=w895) -> ("Gantry Out"=w894:refnum<k24>)  [unwired: 6 in, 2 out]
                                n195 = call "XY Go.vi"("Speed"=w897, "XY In"=w886, "Gantry In"=w894) -> ("Gantry Out"=w893:refnum<k24>)  [unwired: 6 in, 2 out]
                                n196 = call "XY Go.vi"("Speed"=w897, "XY In"=w887, "Gantry In"=w893) -> ("Gantry Out"=w892:refnum<k24>)  [unwired: 6 in, 2 out]
                                n197 = call "XY Go.vi"("Speed"=w897, "XY In"=w888, "Gantry In"=w892) -> ("Gantry Out"=w891:refnum<k24>)  [unwired: 6 in, 2 out]
                                n198 = call "XY Go.vi"("Speed"=w897, "XY In"=w889, "Gantry In"=w891) -> ("Gantry Out"=w890:refnum<k24>)  [unwired: 6 in, 2 out]
                                n199 = Delete From Array(array=w901, length=6, index=0) -> (array with subset deleted=w900:T3)  [unwired: 1 out]
                                }
                                frame True {
                                n200 = case shown="True" w916 {
                                tunnel: w927 -> [w945 w960]
                                tunnel: [w944 w959] -> w926
                                tunnel: w925 -> [w943 w970]
                                tunnel: w924 -> [w942 w969]
                                tunnel: w923 -> [w928 w968]
                                tunnel: w922 -> [w930 w967]
                                tunnel: w921 -> [w929 w966]
                                tunnel: w920 -> [w931 w965]
                                tunnel: w919 -> [w941 w963]
                                tunnel: w918 -> [w940 w962]
                                tunnel: [w933 w961] -> w917
                                tunnel: w915 -> [w932 w964]
                                tunnel: w914 -> [_ w958]
                                tunnel: w913 -> [_ w957]
                                tunnel: w912 -> [_ w956]
                                tunnel: w911 -> [_ w955]
                                tunnel: w910 -> [_ w954]
                                tunnel: w909 -> [_ w953]
                                tunnel: w908 -> [_ w952]
                                tunnel: w907 -> [_ w951]
                                tunnel: w906 -> [_ w950]
                                tunnel: w905 -> [_ w949]
                                tunnel: w904 -> [_ w948]
                                frame False {
                                n201 = call "XY Go.vi"("Speed"=w941, "XY In"=w943, "Gantry In"=w940) -> ("Gantry Out"=w939:refnum<k24>)  [unwired: 6 in, 2 out]
                                n202 = call "XY Go.vi"("Speed"=w941, "XY In"=w942, "Gantry In"=w939) -> ("Gantry Out"=w938:refnum<k24>)  [unwired: 6 in, 2 out]
                                n203 = call "XY Go.vi"("Speed"=w941, "XY In"=w930, "Gantry In"=w938) -> ("Gantry Out"=w937:refnum<k24>)  [unwired: 6 in, 2 out]
                                n204 = call "XY Go.vi"("Speed"=w941, "XY In"=w931, "Gantry In"=w937) -> ("Gantry Out"=w936:refnum<k24>)  [unwired: 6 in, 2 out]
                                n205 = call "XY Go.vi"("Speed"=w941, "XY In"=w928, "Gantry In"=w936) -> ("Gantry Out"=w935:refnum<k24>)  [unwired: 6 in, 2 out]
                                n206 = call "XY Go.vi"("Speed"=w941, "XY In"=w929, "Gantry In"=w935) -> ("Gantry Out"=w934:refnum<k24>)  [unwired: 6 in, 2 out]
                                n207 = call "XY Go.vi"("Speed"=w941, "XY In"=w932, "Gantry In"=w934) -> ("Gantry Out"=w933:refnum<k24>)  [unwired: 6 in, 2 out]
                                n208 = Delete From Array(array=w945, length=7, index=0) -> (array with subset deleted=w944:T3)  [unwired: 1 out]
                                }
                                frame True {
                                n209 = case shown="True" w957 {
                                tunnel: w970 -> [w992 w1012]
                                tunnel: w969 -> [w991 w1011]
                                tunnel: w968 -> [w972 w1010]
                                tunnel: w967 -> [w974 w1009]
                                tunnel: w966 -> [w971 w1008]
                                tunnel: w965 -> [w973 w1007]
                                tunnel: w964 -> [w990 w1006]
                                tunnel: w963 -> [w989 w1004]
                                tunnel: w962 -> [w988 w1003]
                                tunnel: [w980 w1002] -> w961
                                tunnel: w960 -> [w977 w1014]
                                tunnel: [w976 w1013] -> w959
                                tunnel: w958 -> [w975 w1005]
                                tunnel: w956 -> [_ w1001]
                                tunnel: w955 -> [_ w1000]
                                tunnel: w954 -> [_ w999]
                                tunnel: w953 -> [_ w998]
                                tunnel: w952 -> [_ w997]
                                tunnel: w951 -> [_ w996]
                                tunnel: w950 -> [_ w995]
                                tunnel: w949 -> [_ w994]
                                tunnel: w948 -> [_ w993]
                                frame False {
                                n210 = call "XY Go.vi"("Speed"=w989, "XY In"=w992, "Gantry In"=w988) -> ("Gantry Out"=w987:refnum<k24>)  [unwired: 6 in, 2 out]
                                n211 = call "XY Go.vi"("Speed"=w989, "XY In"=w991, "Gantry In"=w987) -> ("Gantry Out"=w986:refnum<k24>)  [unwired: 6 in, 2 out]
                                n212 = call "XY Go.vi"("Speed"=w989, "XY In"=w974, "Gantry In"=w986) -> ("Gantry Out"=w985:refnum<k24>)  [unwired: 6 in, 2 out]
                                n213 = call "XY Go.vi"("Speed"=w989, "XY In"=w973, "Gantry In"=w985) -> ("Gantry Out"=w984:refnum<k24>)  [unwired: 6 in, 2 out]
                                n214 = call "XY Go.vi"("Speed"=w989, "XY In"=w972, "Gantry In"=w984) -> ("Gantry Out"=w983:refnum<k24>)  [unwired: 6 in, 2 out]
                                n215 = call "XY Go.vi"("Speed"=w989, "XY In"=w971, "Gantry In"=w983) -> ("Gantry Out"=w982:refnum<k24>)  [unwired: 6 in, 2 out]
                                n216 = call "XY Go.vi"("Speed"=w989, "XY In"=w990, "Gantry In"=w982) -> ("Gantry Out"=w981:refnum<k24>)  [unwired: 6 in, 2 out]
                                n217 = call "XY Go.vi"("Speed"=w989, "XY In"=w975, "Gantry In"=w981) -> ("Gantry Out"=w980:refnum<k24>)  [unwired: 6 in, 2 out]
                                n218 = Delete From Array(array=w977, length=8, index=0) -> (array with subset deleted=w976:T3)  [unwired: 1 out]
                                }
                                frame True {
                                n219 = case shown="True" w1000 {
                                tunnel: w1014 -> [w1038 w1059]
                                tunnel: [w1037 w1058] -> w1013
                                tunnel: w1012 -> [w1034 w1057]
                                tunnel: w1011 -> [w1033 w1056]
                                tunnel: w1010 -> [w1018 w1055]
                                tunnel: w1009 -> [w1017 w1054]
                                tunnel: w1008 -> [w1016 w1053]
                                tunnel: w1007 -> [w1015 w1052]
                                tunnel: w1006 -> [w1032 w1051]
                                tunnel: w1005 -> [w1031 w1050]
                                tunnel: w1004 -> [w1030 w1048]
                                tunnel: w1003 -> [w1029 w1047]
                                tunnel: [w1020 w1046] -> w1002
                                tunnel: w1001 -> [w1019 w1049]
                                tunnel: w999 -> [_ w1045]
                                tunnel: w998 -> [_ w1044]
                                tunnel: w997 -> [_ w1043]
                                tunnel: w996 -> [_ w1042]
                                tunnel: w995 -> [_ w1041]
                                tunnel: w994 -> [_ w1040]
                                tunnel: w993 -> [_ w1039]
                                frame False {
                                n220 = call "XY Go.vi"("Speed"=w1030, "XY In"=w1034, "Gantry In"=w1029) -> ("Gantry Out"=w1028:refnum<k24>)  [unwired: 6 in, 2 out]
                                n221 = call "XY Go.vi"("Speed"=w1030, "XY In"=w1033, "Gantry In"=w1028) -> ("Gantry Out"=w1027:refnum<k24>)  [unwired: 6 in, 2 out]
                                n222 = call "XY Go.vi"("Speed"=w1030, "XY In"=w1017, "Gantry In"=w1027) -> ("Gantry Out"=w1026:refnum<k24>)  [unwired: 6 in, 2 out]
                                n223 = call "XY Go.vi"("Speed"=w1030, "XY In"=w1015, "Gantry In"=w1026) -> ("Gantry Out"=w1025:refnum<k24>)  [unwired: 6 in, 2 out]
                                n224 = call "XY Go.vi"("Speed"=w1030, "XY In"=w1018, "Gantry In"=w1025) -> ("Gantry Out"=w1024:refnum<k24>)  [unwired: 6 in, 2 out]
                                n225 = call "XY Go.vi"("Speed"=w1030, "XY In"=w1016, "Gantry In"=w1024) -> ("Gantry Out"=w1023:refnum<k24>)  [unwired: 6 in, 2 out]
                                n226 = call "XY Go.vi"("Speed"=w1030, "XY In"=w1032, "Gantry In"=w1023) -> ("Gantry Out"=w1022:refnum<k24>)  [unwired: 6 in, 2 out]
                                n227 = call "XY Go.vi"("Speed"=w1030, "XY In"=w1031, "Gantry In"=w1022) -> ("Gantry Out"=w1021:refnum<k24>)  [unwired: 6 in, 2 out]
                                n228 = call "XY Go.vi"("Speed"=w1030, "XY In"=w1019, "Gantry In"=w1021) -> ("Gantry Out"=w1020:refnum<k24>)  [unwired: 6 in, 2 out]
                                n229 = Delete From Array(array=w1038, length=9, index=0) -> (array with subset deleted=w1037:T3)  [unwired: 1 out]
                                }
                                frame True {
                                n230 = case shown="True" w1044 {
                                tunnel: w1059 -> [w1085 w1105]
                                tunnel: [w1082 w1104] -> w1058
                                tunnel: w1057 -> [w1081 w1101]
                                tunnel: w1056 -> [w1080 w1100]
                                tunnel: w1055 -> [w1063 w1099]
                                tunnel: w1054 -> [w1062 w1098]
                                tunnel: w1053 -> [w1061 w1097]
                                tunnel: w1052 -> [w1060 w1096]
                                tunnel: w1051 -> [w1079 w1095]
                                tunnel: w1050 -> [w1078 w1094]
                                tunnel: w1049 -> [w1077 w1093]
                                tunnel: w1048 -> [w1076 w1091]
                                tunnel: w1047 -> [w1075 w1103]
                                tunnel: [w1065 w1102] -> w1046
                                tunnel: w1045 -> [w1064 w1092]
                                tunnel: w1043 -> [_ w1090]
                                tunnel: w1042 -> [_ w1089]
                                tunnel: w1041 -> [_ w1088]
                                tunnel: w1040 -> [_ w1087]
                                tunnel: w1039 -> [_ w1086]
                                frame False {
                                n231 = call "XY Go.vi"("Speed"=w1076, "XY In"=w1081, "Gantry In"=w1075) -> ("Gantry Out"=w1074:refnum<k24>)  [unwired: 6 in, 2 out]
                                n232 = Delete From Array(array=w1085, length=10, index=0) -> (array with subset deleted=w1082:T3)  [unwired: 1 out]
                                n233 = call "XY Go.vi"("Speed"=w1076, "XY In"=w1080, "Gantry In"=w1074) -> ("Gantry Out"=w1073:refnum<k24>)  [unwired: 6 in, 2 out]
                                n234 = call "XY Go.vi"("Speed"=w1076, "XY In"=w1062, "Gantry In"=w1073) -> ("Gantry Out"=w1072:refnum<k24>)  [unwired: 6 in, 2 out]
                                n235 = call "XY Go.vi"("Speed"=w1076, "XY In"=w1060, "Gantry In"=w1072) -> ("Gantry Out"=w1071:refnum<k24>)  [unwired: 6 in, 2 out]
                                n236 = call "XY Go.vi"("Speed"=w1076, "XY In"=w1063, "Gantry In"=w1071) -> ("Gantry Out"=w1070:refnum<k24>)  [unwired: 6 in, 2 out]
                                n237 = call "XY Go.vi"("Speed"=w1076, "XY In"=w1061, "Gantry In"=w1070) -> ("Gantry Out"=w1069:refnum<k24>)  [unwired: 6 in, 2 out]
                                n238 = call "XY Go.vi"("Speed"=w1076, "XY In"=w1079, "Gantry In"=w1069) -> ("Gantry Out"=w1068:refnum<k24>)  [unwired: 6 in, 2 out]
                                n239 = call "XY Go.vi"("Speed"=w1076, "XY In"=w1078, "Gantry In"=w1068) -> ("Gantry Out"=w1067:refnum<k24>)  [unwired: 6 in, 2 out]
                                n240 = call "XY Go.vi"("Speed"=w1076, "XY In"=w1077, "Gantry In"=w1067) -> ("Gantry Out"=w1066:refnum<k24>)  [unwired: 6 in, 2 out]
                                n241 = call "XY Go.vi"("Speed"=w1076, "XY In"=w1064, "Gantry In"=w1066) -> ("Gantry Out"=w1065:refnum<k24>)  [unwired: 6 in, 2 out]
                                }
                                frame True {
                                n242 = case shown="True" w1089 {
                                tunnel: w1105 -> [w1133 w1152]
                                tunnel: [w1130 w1151] -> w1104
                                tunnel: w1103 -> [w1129 w1139]
                                tunnel: [w1118 w1138] -> w1102
                                tunnel: w1101 -> [w1117 w1150]
                                tunnel: w1100 -> [w1116 w1149]
                                tunnel: w1099 -> [w1110 w1148]
                                tunnel: w1098 -> [w1108 w1147]
                                tunnel: w1097 -> [w1109 w1146]
                                tunnel: w1096 -> [w1111 w1145]
                                tunnel: w1095 -> [w1115 w1144]
                                tunnel: w1094 -> [w1114 w1143]
                                tunnel: w1093 -> [w1106 w1142]
                                tunnel: w1092 -> [w1107 w1141]
                                tunnel: w1091 -> [w1113 w1134]
                                tunnel: w1090 -> [w1112 w1140]
                                tunnel: w1088 -> [_ w1137]
                                tunnel: w1087 -> [_ w1136]
                                tunnel: w1086 -> [_ w1135]
                                frame False {
                                n243 = call "XY Go.vi"("Speed"=w1113, "XY In"=w1117, "Gantry In"=w1129) -> ("Gantry Out"=w1128:refnum<k24>)  [unwired: 6 in, 2 out]
                                n244 = Delete From Array(array=w1133, length=11, index=0) -> (array with subset deleted=w1130:T3)  [unwired: 1 out]
                                n245 = call "XY Go.vi"("Speed"=w1113, "XY In"=w1116, "Gantry In"=w1128) -> ("Gantry Out"=w1127:refnum<k24>)  [unwired: 6 in, 2 out]
                                n246 = call "XY Go.vi"("Speed"=w1113, "XY In"=w1108, "Gantry In"=w1127) -> ("Gantry Out"=w1126:refnum<k24>)  [unwired: 6 in, 2 out]
                                n247 = call "XY Go.vi"("Speed"=w1113, "XY In"=w1111, "Gantry In"=w1126) -> ("Gantry Out"=w1125:refnum<k24>)  [unwired: 6 in, 2 out]
                                n248 = call "XY Go.vi"("Speed"=w1113, "XY In"=w1110, "Gantry In"=w1125) -> ("Gantry Out"=w1124:refnum<k24>)  [unwired: 6 in, 2 out]
                                n249 = call "XY Go.vi"("Speed"=w1113, "XY In"=w1109, "Gantry In"=w1124) -> ("Gantry Out"=w1123:refnum<k24>)  [unwired: 6 in, 2 out]
                                n250 = call "XY Go.vi"("Speed"=w1113, "XY In"=w1115, "Gantry In"=w1123) -> ("Gantry Out"=w1122:refnum<k24>)  [unwired: 6 in, 2 out]
                                n251 = call "XY Go.vi"("Speed"=w1113, "XY In"=w1114, "Gantry In"=w1122) -> ("Gantry Out"=w1121:refnum<k24>)  [unwired: 6 in, 2 out]
                                n252 = call "XY Go.vi"("Speed"=w1113, "XY In"=w1106, "Gantry In"=w1121) -> ("Gantry Out"=w1120:refnum<k24>)  [unwired: 6 in, 2 out]
                                n253 = call "XY Go.vi"("Speed"=w1113, "XY In"=w1107, "Gantry In"=w1120) -> ("Gantry Out"=w1119:refnum<k24>)  [unwired: 6 in, 2 out]
                                n254 = call "XY Go.vi"("Speed"=w1113, "XY In"=w1112, "Gantry In"=w1119) -> ("Gantry Out"=w1118:refnum<k24>)  [unwired: 6 in, 2 out]
                                }
                                frame True {
                                n255 = case shown="True" w1136 {
                                tunnel: w1152 -> [w1181 w1214]
                                tunnel: [w1180 w1213] -> w1151
                                tunnel: w1150 -> [w1179 w1212]
                                tunnel: w1149 -> [w1178 w1211]
                                tunnel: w1148 -> [w1155 w1186]
                                tunnel: w1147 -> [w1153 w1184]
                                tunnel: w1146 -> [w1154 w1187]
                                tunnel: w1145 -> [w1156 w1185]
                                tunnel: w1144 -> [w1177 w1210]
                                tunnel: w1143 -> [w1176 w1209]
                                tunnel: w1142 -> [w1175 w1208]
                                tunnel: w1141 -> [w1174 w1207]
                                tunnel: w1140 -> [w1173 w1206]
                                tunnel: w1139 -> [w1172 w1203]
                                tunnel: [w1160 w1190] -> w1138
                                tunnel: w1137 -> [w1159 w1205]
                                tunnel: w1135 -> [_ w1204]
                                tunnel: w1134 -> [w1157 w1189]
                                frame False {
                                w1158 = FALSE
                                n256 = Delete From Array(array=w1181, length=12, index=0) -> (array with subset deleted=w1180:T3)  [unwired: 1 out]
                                n257 = call "XY Go.vi"("return immediately"=w1158, "Speed"=w1157, "XY In"=w1179, "Gantry In"=w1172) -> ("Gantry Out"=w1171:refnum<k24>)  [unwired: 5 in, 2 out]
                                n258 = call "XY Go.vi"("return immediately"=w1158, "Speed"=w1157, "XY In"=w1178, "Gantry In"=w1171) -> ("Gantry Out"=w1170:refnum<k24>)  [unwired: 5 in, 2 out]
                                n259 = call "XY Go.vi"("return immediately"=w1158, "Speed"=w1157, "XY In"=w1153, "Gantry In"=w1170) -> ("Gantry Out"=w1169:refnum<k24>)  [unwired: 5 in, 2 out]
                                n260 = call "XY Go.vi"("return immediately"=w1158, "Speed"=w1157, "XY In"=w1156, "Gantry In"=w1169) -> ("Gantry Out"=w1168:refnum<k24>)  [unwired: 5 in, 2 out]
                                n261 = call "XY Go.vi"("return immediately"=w1158, "Speed"=w1157, "XY In"=w1155, "Gantry In"=w1168) -> ("Gantry Out"=w1167:refnum<k24>)  [unwired: 5 in, 2 out]
                                n262 = call "XY Go.vi"("return immediately"=w1158, "Speed"=w1157, "XY In"=w1154, "Gantry In"=w1167) -> ("Gantry Out"=w1166:refnum<k24>)  [unwired: 5 in, 2 out]
                                n263 = call "XY Go.vi"("return immediately"=w1158, "Speed"=w1157, "XY In"=w1177, "Gantry In"=w1166) -> ("Gantry Out"=w1165:refnum<k24>)  [unwired: 5 in, 2 out]
                                n264 = call "XY Go.vi"("return immediately"=w1158, "Speed"=w1157, "XY In"=w1176, "Gantry In"=w1165) -> ("Gantry Out"=w1164:refnum<k24>)  [unwired: 5 in, 2 out]
                                n265 = call "XY Go.vi"("return immediately"=w1158, "Speed"=w1157, "XY In"=w1175, "Gantry In"=w1164) -> ("Gantry Out"=w1163:refnum<k24>)  [unwired: 5 in, 2 out]
                                n266 = call "XY Go.vi"("return immediately"=w1158, "Speed"=w1157, "XY In"=w1174, "Gantry In"=w1163) -> ("Gantry Out"=w1162:refnum<k24>)  [unwired: 5 in, 2 out]
                                n267 = call "XY Go.vi"("return immediately"=w1158, "Speed"=w1157, "XY In"=w1173, "Gantry In"=w1162) -> ("Gantry Out"=w1161:refnum<k24>)  [unwired: 5 in, 2 out]
                                n268 = call "XY Go.vi"("return immediately"=w1158, "Speed"=w1157, "XY In"=w1159, "Gantry In"=w1161) -> ("Gantry Out"=w1160:refnum<k24>)  [unwired: 5 in, 2 out]
                                }
                                frame True {
                                w1188 = FALSE
                                n269 = Delete From Array(array=w1214, length=13, index=0) -> (array with subset deleted=w1213:T3)  [unwired: 1 out]
                                n270 = call "XY Go.vi"("return immediately"=w1188, "Speed"=w1189, "XY In"=w1212, "Gantry In"=w1203) -> ("Gantry Out"=w1202:refnum<k24>)  [unwired: 5 in, 2 out]
                                n271 = call "XY Go.vi"("return immediately"=w1188, "Speed"=w1189, "XY In"=w1211, "Gantry In"=w1202) -> ("Gantry Out"=w1201:refnum<k24>)  [unwired: 5 in, 2 out]
                                n272 = call "XY Go.vi"("return immediately"=w1188, "Speed"=w1189, "XY In"=w1184, "Gantry In"=w1201) -> ("Gantry Out"=w1200:refnum<k24>)  [unwired: 5 in, 2 out]
                                n273 = call "XY Go.vi"("return immediately"=w1188, "Speed"=w1189, "XY In"=w1185, "Gantry In"=w1200) -> ("Gantry Out"=w1199:refnum<k24>)  [unwired: 5 in, 2 out]
                                n274 = call "XY Go.vi"("return immediately"=w1188, "Speed"=w1189, "XY In"=w1186, "Gantry In"=w1199) -> ("Gantry Out"=w1198:refnum<k24>)  [unwired: 5 in, 2 out]
                                n275 = call "XY Go.vi"("return immediately"=w1188, "Speed"=w1189, "XY In"=w1187, "Gantry In"=w1198) -> ("Gantry Out"=w1197:refnum<k24>)  [unwired: 5 in, 2 out]
                                n276 = call "XY Go.vi"("return immediately"=w1188, "Speed"=w1189, "XY In"=w1210, "Gantry In"=w1197) -> ("Gantry Out"=w1196:refnum<k24>)  [unwired: 5 in, 2 out]
                                n277 = call "XY Go.vi"("return immediately"=w1188, "Speed"=w1189, "XY In"=w1209, "Gantry In"=w1196) -> ("Gantry Out"=w1195:refnum<k24>)  [unwired: 5 in, 2 out]
                                n278 = call "XY Go.vi"("return immediately"=w1188, "Speed"=w1189, "XY In"=w1208, "Gantry In"=w1195) -> ("Gantry Out"=w1194:refnum<k24>)  [unwired: 5 in, 2 out]
                                n279 = call "XY Go.vi"("return immediately"=w1188, "Speed"=w1189, "XY In"=w1207, "Gantry In"=w1194) -> ("Gantry Out"=w1193:refnum<k24>)  [unwired: 5 in, 2 out]
                                n280 = call "XY Go.vi"("return immediately"=w1188, "Speed"=w1189, "XY In"=w1206, "Gantry In"=w1193) -> ("Gantry Out"=w1192:refnum<k24>)  [unwired: 5 in, 2 out]
                                n281 = call "XY Go.vi"("return immediately"=w1188, "Speed"=w1189, "XY In"=w1205, "Gantry In"=w1192) -> ("Gantry Out"=w1191:refnum<k24>)  [unwired: 5 in, 2 out]
                                n282 = call "XY Go.vi"("return immediately"=w1188, "Speed"=w1189, "XY In"=w1204, "Gantry In"=w1191) -> ("Gantry Out"=w1190:refnum<k24>)  [unwired: 5 in, 2 out]
                                }
                                }
                                }
                                }
                                }
                                }
                                }
                                }
                                }
                                }
                                }
                                }
                                }
                                }
                                }
                                }
                                }
                              }
                            }
                          }
                        }
                      }
                    }
                  }
                  n283 = flat-sequence {
                    tunnel: [w1217] -> w686
                    tunnel: [w1221] -> w683
                    tunnel: [w1220] -> w680
                    tunnel: w685 -> [w1222]
                    tunnel: w682 -> [w1221]
                    tunnel: w679 -> [w1220]
                    tunnel: w674 -> [w1218]
                    tunnel: w647 -> [w1217]
                    tunnel: [w1226] -> w687
                    tunnel: w686 -> [w1225]
                    tunnel: [w1224] -> w684
                    tunnel: w683 -> [w1224]
                    tunnel: [w1223] -> w681
                    tunnel: w680 -> [w1223]
                    frame #0 {
                      n284 = Subtract(x=w1222, y=w1218) -> (x-y=w1219:i32)
                      n285 = Wait (ms)(milliseconds to wait=w1219) -> ()  [unwired: 1 out]
                    }
                    frame #1 {
                      n286 = call "Dispense.vi"("Dispenser In"=w1225) -> ("Dispenser Out"=w1226:refnum<visa-resource-name>)  [unwired: 9 in, 1 out]
                    }
                  }
                }
                frame #3 {
                  n287 = Negate(x=w1231) -> (-x=w1230:dbl)
                  n288 = call "Z Go.vi"("Increment"=TRUE, "Return Immediately"=FALSE, "Speed In"=w1229, "Position In"=w1230, "Gantry In"=w1232) -> ("Gantry Out"=w1234:refnum<k24>)  [unwired: 3 in, 3 out]
                }
              }
            }
            frame "Arc" {
              n289 = flat-sequence {
                tunnel: [w1281] -> w1273
                tunnel: w1265 -> [w1274]
                tunnel: w1264 -> [w1280]
                tunnel: w1236 -> [w1279]
                tunnel: w1263 -> [w1278]
                tunnel: [w1277] -> w1251
                tunnel: w1250 -> [w1276]
                tunnel: w1249 -> [w1275]
                tunnel: w1273 -> [w1307]
                tunnel: [w1308] -> w1272
                tunnel: [w1304] -> w1271
                tunnel: [w1301] -> w1270
                tunnel: [w1298] -> w1269
                tunnel: w1262 -> [w1297]
                tunnel: w1261 -> [w1296]
                tunnel: w1260 -> [w1295]
                tunnel: w1259 -> [w1294]
                tunnel: w1251 -> [w1293]
                tunnel: w1272 -> [w1351]
                tunnel: [w1352] -> w1268
                tunnel: w1271 -> [w1342]
                tunnel: w1270 -> [w1355]
                tunnel: [w1355] -> w1267
                tunnel: w1269 -> [w1354]
                tunnel: [w1354] -> w1266
                tunnel: w1235 -> [w1345]
                tunnel: w1258 -> [w1344]
                tunnel: w1257 -> [w1346]
                tunnel: w1256 -> [w1348]
                tunnel: w1255 -> [w1353]
                tunnel: [w1343] -> w1252
                tunnel: w1248 -> [w1349]
                tunnel: w1247 -> [w1341]
                tunnel: w1246 -> [w1340]
                tunnel: w1245 -> [w1339]
                tunnel: w1236 -> [w1338]
                tunnel: w1244 -> [w1337]
                tunnel: w1243 -> [w1336]
                tunnel: w1242 -> [w1335]
                tunnel: w1241 -> [w1334]
                tunnel: w1240 -> [w1333]
                tunnel: w1239 -> [w1332]
                tunnel: [w1331] -> w1238
                tunnel: w1237 -> [w1330]
                tunnel: [w1464] -> w1254
                tunnel: w1268 -> [w1463]
                tunnel: [w1463] -> w1253
                tunnel: w1267 -> [w1461]
                tunnel: w1266 -> [w1459]
                tunnel: w1252 -> [w1462]
                frame #0 {
                  n290 = case shown="False" w1274 {
                    tunnel: [w1286 w1290] -> w1281
                    tunnel: w1280 -> [w1285 w1289]
                    tunnel: w1279 -> [w1284 w1288]
                    tunnel: w1278 -> [w1283 _]
                    frame False {
                      n291 = call "XY Go.vi"("return immediately"=FALSE, "Speed"=w1283, "XY In"=w1284, "Gantry In"=w1285) -> ("Gantry Out"=w1286:refnum<k24>)  [unwired: 5 in, 2 out]
                    }
                    frame True {
                      n292 = call "ClearXYZTheta Go.vi"("Speed"=300.0, "XYZTheta In"=w1288, "Gantry In"=w1289) -> ("Gantry Out"=w1290:refnum<k24>)  [unwired: 6 in, 2 out]
                    }
                  }
                  n293 = call "Pressure.vi"("Pressure"=w1275, "VISA resource name"=w1276) -> ("VISA resource name out"=w1277:refnum<visa-resource-name>)  [unwired: 8 in, 1 out]
                }
                frame #1 {
                  n294 = flat-sequence {
                    tunnel: w1307 -> [w1317]
                    tunnel: [w1315] -> w1306
                    tunnel: [w1314] -> w1303
                    tunnel: [w1313] -> w1302
                    tunnel: w1295 -> [w1312]
                    tunnel: w1294 -> [w1311]
                    tunnel: w1293 -> [w1309]
                    tunnel: [w1309] -> w1292
                    tunnel: w1306 -> [w1324]
                    tunnel: [w1324] -> w1305
                    tunnel: w1303 -> [w1323]
                    tunnel: w1302 -> [w1322]
                    tunnel: [w1323] -> w1300
                    tunnel: [w1322] -> w1299
                    tunnel: w1297 -> [w1321]
                    tunnel: w1296 -> [w1320]
                    tunnel: w1292 -> [w1319]
                    tunnel: [w1319] -> w1291
                    tunnel: [w1329] -> w1308
                    tunnel: w1305 -> [w1328]
                    tunnel: [w1328] -> w1304
                    tunnel: [w1327] -> w1301
                    tunnel: w1300 -> [w1327]
                    tunnel: w1299 -> [w1326]
                    tunnel: [w1326] -> _
                    tunnel: [w1326] -> w1298
                    tunnel: w1291 -> [w1325]
                    frame #0 {
                      n295 = call "Z Go.vi"("Increment"=TRUE, "Return Immediately"=TRUE, "Speed In"=w1311, "Position In"=w1312, "Gantry In"=w1317) -> ("Speed Out"=w1313:dbl, "Position Out"=w1314:dbl, "Gantry Out"=w1315:refnum<k24>)  [unwired: 3 in, 1 out]
                    }
                    frame #1 {
                      n296 = Subtract(x=w1321, y=w1320) -> (x-y=w1318:i32)
                      n297 = Wait (ms)(milliseconds to wait=w1318) -> ()  [unwired: 1 out]
                    }
                    frame #2 {
                      n298 = call "Dispense.vi"("Dispenser In"=w1325) -> ("Dispenser Out"=w1329:refnum<visa-resource-name>)  [unwired: 9 in, 1 out]
                    }
                  }
                }
                frame #2 {
                  n299 = flat-sequence {
                    tunnel: [w1452] -> w1350
                    tunnel: w1353 -> [w1454]
                    tunnel: w1351 -> [w1452]
                    tunnel: w1349 -> [w1451]
                    tunnel: [w1456] -> w1352
                    tunnel: w1350 -> [w1455]
                    frame #0 {
                      n300 = Subtract(x=w1454, y=w1451) -> (x-y=w1453:i32)
                      n301 = Wait (ms)(milliseconds to wait=w1453) -> ()  [unwired: 1 out]
                    }
                    frame #1 {
                      n302 = call "Dispense.vi"("Dispenser In"=w1455) -> ("Dispenser Out"=w1456:refnum<visa-resource-name>)  [unwired: 9 in, 1 out]
                    }
                  }
                  n303 = case shown="True" w1335 {
                    tunnel: w1348 -> [w1366 w1381]
                    tunnel: FALSE ("return immediately") -> [w1365 _]
                    tunnel: w1346 -> [w1364 w1380]
                    tunnel: w1345 -> [w1363 w1382]
                    tunnel: w1344 -> [w1362 w1383]
                    tunnel: [w1361 w1370] -> w1343
                    tunnel: w1342 -> [w1360 w1371]
                    tunnel: w1341 -> [_ w1379]
                    tunnel: w1340 -> [_ w1378]
                    tunnel: w1339 -> [_ w1377]
                    tunnel: w1338 -> [_ w1376]
                    tunnel: w1337 -> [_ w1375]
                    tunnel: w1336 -> [_ w1374]
                    tunnel: w1334 -> [_ w1373]
                    tunnel: w1333 -> [_ w1372]
                    tunnel: w1332 -> [w1359 w1369]
                    tunnel: [w1356 w1368] -> w1331
                    tunnel: w1330 -> [_ w1367]
                    frame False {
                      n304 = call "Circular.vi"("Direction"=w1366, "return immediately"=w1365, "Speed"=w1364, "XY End"=w1363, "XY Center"=w1362, "Gantry In"=w1360) -> ("Gantry Out"=w1361:refnum<k24>)  [unwired: 4 in, 1 out]
                      n305 = Delete From Array(array=w1359, length=1, index=0) -> (array with subset deleted=w1356:T3)  [unwired: 1 out]
                    }
                    frame True {
                      n306 = case shown="True" w1373 {
                        tunnel: w1383 -> [w1397 w1411]
                        tunnel: w1382 -> [w1396 w1410]
                        tunnel: w1381 -> [w1395 w1401]
                        tunnel: w1380 -> [w1394 w1402]
                        tunnel: w1379 -> [w1392 w1412]
                        tunnel: w1378 -> [w1391 w1413]
                        tunnel: w1377 -> [_ w1409]
                        tunnel: w1376 -> [_ w1408]
                        tunnel: w1375 -> [_ w1407]
                        tunnel: w1374 -> [_ w1406]
                        tunnel: w1372 -> [_ w1405]
                        tunnel: w1371 -> [w1390 w1404]
                        tunnel: [w1388 w1403] -> w1370
                        tunnel: w1369 -> [w1387 w1400]
                        tunnel: [w1386 w1399] -> w1368
                        tunnel: w1367 -> [_ w1398]
                        frame False {
                          w1393 = FALSE
                          n307 = call "Circular.vi"("Direction"=w1395, "return immediately"=w1393, "Speed"=w1394, "XY End"=w1396, "XY Center"=w1397, "Gantry In"=w1390) -> ("Gantry Out"=w1389:refnum<k24>)  [unwired: 4 in, 1 out]
                          n308 = call "Circular.vi"("Direction"=w1395, "return immediately"=w1393, "Speed"=w1394, "XY End"=w1392, "XY Center"=w1391, "Gantry In"=w1389) -> ("Gantry Out"=w1388:refnum<k24>)  [unwired: 4 in, 1 out]
                          n309 = Delete From Array(array=w1387, length=2, index=0) -> (array with subset deleted=w1386:T3)  [unwired: 1 out]
                        }
                        frame True {
                          n310 = case shown="True" w1405 {
                            tunnel: w1413 -> [w1429 w1450]
                            tunnel: w1412 -> [w1426 w1449]
                            tunnel: w1411 -> [w1428 w1448]
                            tunnel: w1410 -> [w1427 w1447]
                            tunnel: w1409 -> [w1430 w1446]
                            tunnel: w1408 -> [_ _]
                            tunnel: w1407 -> [_ w1445]
                            tunnel: w1406 -> [_ w1444]
                            tunnel: w1404 -> [w1425 w1443]
                            tunnel: [w1422 w1439] -> w1403
                            tunnel: w1402 -> [w1421 w1438]
                            tunnel: w1401 -> [w1420 w1437]
                            tunnel: w1400 -> [w1418 w1435]
                            tunnel: [w1417 w1434] -> w1399
                            tunnel: w1398 -> [w1414 w1431]
                            frame False {
                              w1419 = FALSE
                              n311 = call "Circular.vi"("Direction"=w1420, "return immediately"=w1419, "Speed"=w1421, "XY End"=w1427, "XY Center"=w1428, "Gantry In"=w1425) -> ("Gantry Out"=w1424:refnum<k24>)  [unwired: 4 in, 1 out]
                              n312 = call "Circular.vi"("Direction"=w1420, "return immediately"=w1419, "Speed"=w1421, "XY End"=w1426, "XY Center"=w1429, "Gantry In"=w1424) -> ("Gantry Out"=w1423:refnum<k24>)  [unwired: 4 in, 1 out]
                              n313 = call "Circular.vi"("Direction"=w1420, "return immediately"=w1419, "Speed"=w1421, "XY End"=w1414, "XY Center"=w1430, "Gantry In"=w1423) -> ("Gantry Out"=w1422:refnum<k24>)  [unwired: 4 in, 1 out]
                              n314 = Delete From Array(array=w1418, length=3, index=0) -> (array with subset deleted=w1417:T3)  [unwired: 1 out]
                            }
                            frame True {
                              w1436 = FALSE
                              n315 = Delete From Array(array=w1435, length=4, index=0) -> (array with subset deleted=w1434:T3)  [unwired: 1 out]
                              n316 = call "Circular.vi"("Direction"=w1437, "return immediately"=w1436, "Speed"=w1438, "XY End"=w1447, "XY Center"=w1448, "Gantry In"=w1443) -> ("Gantry Out"=w1442:refnum<k24>)  [unwired: 4 in, 1 out]
                              n317 = call "Circular.vi"("Direction"=w1437, "return immediately"=w1436, "Speed"=w1438, "XY End"=w1449, "XY Center"=w1450, "Gantry In"=w1442) -> ("Gantry Out"=w1441:refnum<k24>)  [unwired: 4 in, 1 out]
                              n318 = call "Circular.vi"("Direction"=w1437, "return immediately"=w1436, "Speed"=w1438, "XY End"=w1431, "XY Center"=w1446, "Gantry In"=w1441) -> ("Gantry Out"=w1440:refnum<k24>)  [unwired: 4 in, 1 out]
                              n319 = call "Circular.vi"("Direction"=w1437, "return immediately"=w1436, "Speed"=w1438, "XY End"=w1444, "XY Center"=w1445, "Gantry In"=w1440) -> ("Gantry Out"=w1439:refnum<k24>)  [unwired: 4 in, 1 out]
                            }
                          }
                        }
                      }
                    }
                  }
                }
                frame #3 {
                  n320 = Negate(x=w1461) -> (-x=w1460:dbl)
                  n321 = call "Z Go.vi"("Increment"=TRUE, "Return Immediately"=FALSE, "Speed In"=w1459, "Position In"=w1460, "Gantry In"=w1462) -> ("Gantry Out"=w1464:refnum<k24>)  [unwired: 3 in, 3 out]
                }
              }
            }
          }
          n322 = Array Size(array=w128) -> (size(s)=w129:i32)
          n323 = Equal To 0?(x=w129) -> (x = 0?=w130:bool)
        }
        n324 = in-place-cluster #1("Gantry"=w25, "Dispenser"=w21) -> (w11:T2)
      }
    }
    frame Error {
    }
  }
  "error out" <- w3
  "Sensor Dispense out" <- w6
  "Control Out" <- w4
